vi "Periodic Tasks.vi"(8 "error in":errorcluster) -> ()   [LabVIEW 2020]
doc: "This VI runs in parallel to other tasks. It can contain as many user-defined periodic loops as you need. These can carry out PID or other sorts of timed response."
uses:
  <vilib>/Rock Robotics/WPI/ThirdParty/Phoenix-LabVIEW/Motor Controller/Controls/CTRE_Phoenix_MotorControl_TalonFXMotorControllerConfigurables.ctl
  <vilib>/Rock Robotics/WPI/ThirdParty/Phoenix-LabVIEW/Motor Controller/Controls/CTRE_Phoenix_MotorControl_BaseConfigurables.ctl
  <vilib>/Rock Robotics/WPI/ThirdParty/Phoenix-LabVIEW/Motor Controller/Controls/CTRE_Phoenix_MotorControl_VelocityMeasurementPeriod.ctl
  <vilib>/Rock Robotics/WPI/ThirdParty/Phoenix-LabVIEW/Motor Controller/Controls/CTRE_Phoenix_MotorControl_SlotStructure.ctl
  <vilib>/Rock Robotics/WPI/ThirdParty/Phoenix-LabVIEW/Motor Controller/Controls/CTRE_Phoenix_MotorControl_FilterStruct.ctl
  <vilib>/Rock Robotics/WPI/ThirdParty/Phoenix-LabVIEW/Motor Controller/Controls/CTRE_Phoenix_MotorControl_RemoteSourceType.ctl
  <vilib>/Rock Robotics/WPI/ThirdParty/Phoenix-LabVIEW/Controls/CTRE_Phoenix_CustomParamConfiguration.ctl
  <vilib>/Rock Robotics/WPI/ThirdParty/Phoenix-LabVIEW/Motor Controller/Controls/CTRE_Phoenix_MotorControl_FeedbackDevice_TalonFX.ctl
  <vilib>/Rock Robotics/WPI/ThirdParty/Phoenix-LabVIEW/Motor Controller/Controls/CTRE_Phoenix_MotorControl_LimitSwitchNormal.ctl
  <vilib>/Rock Robotics/WPI/ThirdParty/Phoenix-LabVIEW/Motor Controller/Controls/CTRE_Phoenix_MotorControl_LimitSwitchSource_Local.ctl
  <vilib>/Rock Robotics/WPI/ThirdParty/Phoenix-LabVIEW/Motor Controller/Controls/CTRE_Phoenix_MotorControl_SupplyCurrentLimitConfiguration.ctl
  <vilib>/Rock Robotics/WPI/ThirdParty/Phoenix-LabVIEW/Motor Controller/Controls/CTRE_Phoenix_MotorControl_StatorCurrentLimitConfiguration.ctl
  <vilib>/Rock Robotics/WPI/ThirdParty/Phoenix-LabVIEW/Motor Controller/Controls/CTRE_Phoenix_MotorControl_MotorCommutation_TalonFX.ctl
  <vilib>/Rock Robotics/WPI/ThirdParty/Phoenix-LabVIEW/CANCoder/Controls/CTRE_Phoenix_CANcoder_AbsoluteSensorRange.ctl
  <vilib>/Rock Robotics/WPI/ThirdParty/Phoenix-LabVIEW/CANCoder/Controls/CTRE_Phoenix_CANcoder_SensorInitializationStrategy.ctl
  <vilib>/Rock Robotics/WPI/ThirdParty/REV Robotics/REVLib/Typedef/Spark MAX Limit Direction.ctl
  <vilib>/Rock Robotics/WPI/Solenoid/WPI_SolenoidValue.ctl
  <vilib>/Rock Robotics/WPI/ThirdParty/Phoenix-LabVIEW/Motor Controller/Controls/CTRE_Phoenix_MotorControl_ControlMode.ctl
  <vilib>/Rock Robotics/WPI/DriverStation/WPI_DriverStationRobotMode2.ctl
  <vilib>/Rock Robotics/WPI/DriverStation/WPI_DriverStationAllianceInfo.ctl
  <vilib>/Rock Robotics/WPI/ThirdParty/Phoenix-LabVIEW/Motor Controller/Controls/CTRE_Phoenix_MotorControl_TalonFXInvertType.ctl
  <vilib>/Rock Robotics/WPI/ThirdParty/Phoenix-LabVIEW/Motor Controller/Controls/CTRE_Phoenix_MotorControl_NeutralMode.ctl
  <vilib>/Rock Robotics/WPI/Utilities/WPI_GetSetVariantRefNum.vi
  Robot Global Data.vi
  <vilib>/Rock Robotics/WPI/RobotDrive/WPI_RobotDriveArcadeDrive_Standard(NoSaturation).vi
  <vilib>/Rock Robotics/WPI/ThirdParty/Phoenix-LabVIEW/Motor Controller/Sensor/CTRE_Phoenix_MotorControl_SetIntegratedSensorPosition_TalonFX.vi
  <vilib>/Rock Robotics/WPI/ThirdParty/Phoenix-LabVIEW/Motor Controller/Get/CTRE_Phoenix_MotorController_GetSelectedSensorData.vi
  <vilib>/addons/control/pid/pid.llb/PID (DBL).vi
  <vilib>/Rock Robotics/WPI/Solenoid/WPI_SolenoidSetEnum.vi
  <vilib>/Rock Robotics/WPI/ThirdParty/Phoenix-LabVIEW/Motor Controller/Get/CTRE_Phoenix_MotorController_GetGeneralStatus.vi
  <vilib>/Rock Robotics/Network Tables/NT Read Number.vi
  <vilib>/Rock Robotics/Network Tables/NT Write Number.vi
  <vilib>/Rock Robotics/Network Tables/NT Write String.vi
  <vilib>/express/express arith-compare/Formula/XNode/ExpressFormulaBlockNode.xnode
  <vilib>/FRC Team #3937/Memory Library/memLib.lvlib
  <vilib>/addons/control/pid/NI_PID_pid.lvlib
panel:
  in  "DriveConfig":T1={"Base Configurables"={"openLoopRamp"=0.5, "closedLoopRamp"=0.0, "peakOutputForward"=0.7, "peakOutputReverse"=-0.7, "nominalOutputForward"=0.0, "nominalOutputReverse"=0.0, "neutralDeadband"=0.04, "voltageCompSaturation"=0.0, "voltageMeasurementFilter"=32, "velocityMeasurementPeriod"=100, "velocityMeasurementWindow"=64, "forwardSoftLimitThreshold"=0, "reverseSoftLimitThreshold"=0, "forwardSoftLimitEnable"=FALSE, "reverseSoftLimitEnable"=FALSE, "slot0"={"P"=0.0, "I"=0.0, "D"=0.0, "F"=0.0, "integralZone"=0.0, "allowableClosedLoopError"=0, "maxIntegralAccumulator"=0.0, "closedLoopPeakOutput"=1.0, "closedLoopPeriod"=1}, "slot1"={"P"=0.0, "I"=0.0, "D"=0.0, "F"=0.0, "integralZone"=0.0, "allowableClosedLoopError"=0, "maxIntegralAccumulator"=0.0, "closedLoopPeakOutput"=1.0, "closedLoopPeriod"=1}, "slot2"={"P"=0.0, "I"=0.0, "D"=0.0, "F"=0.0, "integralZone"=0.0, "allowableClosedLoopError"=0, "maxIntegralAccumulator"=0.0, "closedLoopPeakOutput"=1.0, "closedLoopPeriod"=1}, "slot3"={"P"=0.0, "I"=0.0, "D"=0.0, "F"=0.0, "integralZone"=0.0, "allowableClosedLoopError"=0, "maxIntegralAccumulator"=0.0, "closedLoopPeakOutput"=1.0, "closedLoopPeriod"=1}, "auxPIDPolarity"=FALSE, "remoteFilter0"={"remoteSensorDeviceID"=0, "remoteSensorSource"=enum."Off"}, "remoteFilter1"={"remoteSensorDeviceID"=0, "remoteSensorSource"=enum."Off"}, "motionCruiseVelocity"=0, "motionAcceleration"=0, "motionProfileTrajectoryPeriod"=0, "feedbackNotContinuous"=FALSE, "remoteSensorClosedLoopDisableNeutralOnLOS"=FALSE, "clearPositionOnLimitF"=FALSE, "clearPositionOnLimitR"=FALSE, "clearPositionOnQuadIdx"=FALSE, "limitSwitchDisableNeutralOnLOS"=FALSE, "softLimitDisableNeutralOnLOS"=FALSE, "pulseWidthPeriod_EdgesPerRot"=1, "pulseWidthPeriod_FilterWindowSz"=1, "customParam"={"customParam0"=0, "customParam1"=0}, "trajectoryInterpolationEnable"=TRUE}, "primaryPID"={"selectedFeedbackCoefficient"=1.0, "selectedFeedbackSensor"=1}, "auxiliaryPID"={"selectedFeedbackCoefficient"=1.0, "selectedFeedbackSensor"=1}, "forwardLimitSwitchNormal"=enum."Normally Open", "reverseLimitSwitchNormal"=enum."Normally Open", "forwardLimitSwitchDeviceID"=0, "reverseLimitSwitchDeviceID"=0, "forwardLimitSwitchSource"=enum."Feedback Connector", "reverseLimitSwitchSource"=enum."Feedback Connector", "sum0Term"=1, "sum1Term"=1, "diff0Term"=1, "diff1Term"=1, "Supply Current Limit Configuration"={"Enable?"=FALSE, "Current Limit"=0.0, "Threshold Current"=0.0, "Threshold Time"=0.0}, "Stator Current Limit Configuration"={"Enable?"=FALSE, "Current Limit"=0.0, "Threshold Current"=0.0, "Threshold Time"=0.0}, "Motor Commutation"=enum."Trapezoidal", "Absolute Sensor Range"=enum."Unsigned [0 to 360)", "Integrated Sensor Offset (Degrees)"=0.0, "Sensor Initialization Strategy"=enum."Boot To Zero"} {"diff1Term" items=["Integrated Sensor"=1, "Sensor Sum (S0 + S1)"=9, "Sensor Difference (D0 - D1)"=10, "Remote Source 0"=11, "Remote Source 1"=12, "None"=14, "Software Emulated"=15]; "diff0Term" items=["Integrated Sensor"=1, "Sensor Sum (S0 + S1)"=9, "Sensor Difference (D0 - D1)"=10, "Remote Source 0"=11, "Remote Source 1"=12, "None"=14, "Software Emulated"=15]; "sum1Term" items=["Integrated Sensor"=1, "Sensor Sum (S0 + S1)"=9, "Sensor Difference (D0 - D1)"=10, "Remote Source 0"=11, "Remote Source 1"=12, "None"=14, "Software Emulated"=15]; "sum0Term" items=["Integrated Sensor"=1, "Sensor Sum (S0 + S1)"=9, "Sensor Difference (D0 - D1)"=10, "Remote Source 0"=11, "Remote Source 1"=12, "None"=14, "Software Emulated"=15]; "auxiliaryPID"."selectedFeedbackSensor" items=["Integrated Sensor"=1, "Sensor Sum (S0 + S1)"=9, "Sensor Difference (D0 - D1)"=10, "Remote Source 0"=11, "Remote Source 1"=12, "None"=14, "Software Emulated"=15]; "primaryPID"."selectedFeedbackSensor" items=["Integrated Sensor"=1, "Sensor Sum (S0 + S1)"=9, "Sensor Difference (D0 - D1)"=10, "Remote Source 0"=11, "Remote Source 1"=12, "None"=14, "Software Emulated"=15]; "Base Configurables"."velocityMeasurementPeriod" items=["Period_1ms"=1, "Period_2ms"=2, "Period_5ms"=5, "Period_10ms"=10, "Period_20ms"=20, "Period_25ms"=25, "Period_50ms"=50, "Period_100ms"=100]}
  in  "ShootConfig1":T1={"Base Configurables"={"openLoopRamp"=0.0, "closedLoopRamp"=0.0, "peakOutputForward"=1.0, "peakOutputReverse"=0.0, "nominalOutputForward"=0.0, "nominalOutputReverse"=0.0, "neutralDeadband"=0.04, "voltageCompSaturation"=0.0, "voltageMeasurementFilter"=32, "velocityMeasurementPeriod"=100, "velocityMeasurementWindow"=64, "forwardSoftLimitThreshold"=0, "reverseSoftLimitThreshold"=0, "forwardSoftLimitEnable"=FALSE, "reverseSoftLimitEnable"=FALSE, "slot0"={"P"=0.32, "I"=0.0, "D"=45.0, "F"=0.047, "integralZone"=0.0, "allowableClosedLoopError"=0, "maxIntegralAccumulator"=0.0, "closedLoopPeakOutput"=1.0, "closedLoopPeriod"=1}, "slot1"={"P"=0.0, "I"=0.0, "D"=0.0, "F"=0.0, "integralZone"=0.0, "allowableClosedLoopError"=0, "maxIntegralAccumulator"=0.0, "closedLoopPeakOutput"=1.0, "closedLoopPeriod"=1}, "slot2"={"P"=0.0, "I"=0.0, "D"=0.0, "F"=0.0, "integralZone"=0.0, "allowableClosedLoopError"=0, "maxIntegralAccumulator"=0.0, "closedLoopPeakOutput"=1.0, "closedLoopPeriod"=1}, "slot3"={"P"=0.0, "I"=0.0, "D"=0.0, "F"=0.0, "integralZone"=0.0, "allowableClosedLoopError"=0, "maxIntegralAccumulator"=0.0, "closedLoopPeakOutput"=1.0, "closedLoopPeriod"=1}, "auxPIDPolarity"=FALSE, "remoteFilter0"={"remoteSensorDeviceID"=0, "remoteSensorSource"=enum."Off"}, "remoteFilter1"={"remoteSensorDeviceID"=0, "remoteSensorSource"=enum."Off"}, "motionCruiseVelocity"=0, "motionAcceleration"=0, "motionProfileTrajectoryPeriod"=0, "feedbackNotContinuous"=FALSE, "remoteSensorClosedLoopDisableNeutralOnLOS"=FALSE, "clearPositionOnLimitF"=FALSE, "clearPositionOnLimitR"=FALSE, "clearPositionOnQuadIdx"=FALSE, "limitSwitchDisableNeutralOnLOS"=FALSE, "softLimitDisableNeutralOnLOS"=FALSE, "pulseWidthPeriod_EdgesPerRot"=1, "pulseWidthPeriod_FilterWindowSz"=1, "customParam"={"customParam0"=0, "customParam1"=0}, "trajectoryInterpolationEnable"=TRUE}, "primaryPID"={"selectedFeedbackCoefficient"=1.0, "selectedFeedbackSensor"=1}, "auxiliaryPID"={"selectedFeedbackCoefficient"=1.0, "selectedFeedbackSensor"=1}, "forwardLimitSwitchNormal"=enum."Normally Open", "reverseLimitSwitchNormal"=enum."Normally Open", "forwardLimitSwitchDeviceID"=0, "reverseLimitSwitchDeviceID"=0, "forwardLimitSwitchSource"=enum."Feedback Connector", "reverseLimitSwitchSource"=enum."Feedback Connector", "sum0Term"=1, "sum1Term"=1, "diff0Term"=1, "diff1Term"=1, "Supply Current Limit Configuration"={"Enable?"=FALSE, "Current Limit"=0.0, "Threshold Current"=0.0, "Threshold Time"=0.0}, "Stator Current Limit Configuration"={"Enable?"=FALSE, "Current Limit"=0.0, "Threshold Current"=0.0, "Threshold Time"=0.0}, "Motor Commutation"=enum."Trapezoidal", "Absolute Sensor Range"=enum."Unsigned [0 to 360)", "Integrated Sensor Offset (Degrees)"=0.0, "Sensor Initialization Strategy"=enum."Boot To Zero"} {"diff1Term" items=["Integrated Sensor"=1, "Sensor Sum (S0 + S1)"=9, "Sensor Difference (D0 - D1)"=10, "Remote Source 0"=11, "Remote Source 1"=12, "None"=14, "Software Emulated"=15]; "diff0Term" items=["Integrated Sensor"=1, "Sensor Sum (S0 + S1)"=9, "Sensor Difference (D0 - D1)"=10, "Remote Source 0"=11, "Remote Source 1"=12, "None"=14, "Software Emulated"=15]; "sum1Term" items=["Integrated Sensor"=1, "Sensor Sum (S0 + S1)"=9, "Sensor Difference (D0 - D1)"=10, "Remote Source 0"=11, "Remote Source 1"=12, "None"=14, "Software Emulated"=15]; "sum0Term" items=["Integrated Sensor"=1, "Sensor Sum (S0 + S1)"=9, "Sensor Difference (D0 - D1)"=10, "Remote Source 0"=11, "Remote Source 1"=12, "None"=14, "Software Emulated"=15]; "auxiliaryPID"."selectedFeedbackSensor" items=["Integrated Sensor"=1, "Sensor Sum (S0 + S1)"=9, "Sensor Difference (D0 - D1)"=10, "Remote Source 0"=11, "Remote Source 1"=12, "None"=14, "Software Emulated"=15]; "primaryPID"."selectedFeedbackSensor" items=["Integrated Sensor"=1, "Sensor Sum (S0 + S1)"=9, "Sensor Difference (D0 - D1)"=10, "Remote Source 0"=11, "Remote Source 1"=12, "None"=14, "Software Emulated"=15]; "Base Configurables"."velocityMeasurementPeriod" items=["Period_1ms"=1, "Period_2ms"=2, "Period_5ms"=5, "Period_10ms"=10, "Period_20ms"=20, "Period_25ms"=25, "Period_50ms"=50, "Period_100ms"=100]}
  in  "ShootConfig2":T1={"Base Configurables"={"openLoopRamp"=0.0, "closedLoopRamp"=0.0, "peakOutputForward"=1.0, "peakOutputReverse"=0.0, "nominalOutputForward"=0.0, "nominalOutputReverse"=0.0, "neutralDeadband"=0.04, "voltageCompSaturation"=0.0, "voltageMeasurementFilter"=32, "velocityMeasurementPeriod"=100, "velocityMeasurementWindow"=64, "forwardSoftLimitThreshold"=0, "reverseSoftLimitThreshold"=0, "forwardSoftLimitEnable"=FALSE, "reverseSoftLimitEnable"=FALSE, "slot0"={"P"=0.32, "I"=0.0, "D"=45.0, "F"=0.0475, "integralZone"=0.0, "allowableClosedLoopError"=0, "maxIntegralAccumulator"=0.0, "closedLoopPeakOutput"=1.0, "closedLoopPeriod"=1}, "slot1"={"P"=0.0, "I"=0.0, "D"=0.0, "F"=0.0, "integralZone"=0.0, "allowableClosedLoopError"=0, "maxIntegralAccumulator"=0.0, "closedLoopPeakOutput"=1.0, "closedLoopPeriod"=1}, "slot2"={"P"=0.0, "I"=0.0, "D"=0.0, "F"=0.0, "integralZone"=0.0, "allowableClosedLoopError"=0, "maxIntegralAccumulator"=0.0, "closedLoopPeakOutput"=1.0, "closedLoopPeriod"=1}, "slot3"={"P"=0.0, "I"=0.0, "D"=0.0, "F"=0.0, "integralZone"=0.0, "allowableClosedLoopError"=0, "maxIntegralAccumulator"=0.0, "closedLoopPeakOutput"=1.0, "closedLoopPeriod"=1}, "auxPIDPolarity"=FALSE, "remoteFilter0"={"remoteSensorDeviceID"=0, "remoteSensorSource"=enum."Off"}, "remoteFilter1"={"remoteSensorDeviceID"=0, "remoteSensorSource"=enum."Off"}, "motionCruiseVelocity"=0, "motionAcceleration"=0, "motionProfileTrajectoryPeriod"=0, "feedbackNotContinuous"=FALSE, "remoteSensorClosedLoopDisableNeutralOnLOS"=FALSE, "clearPositionOnLimitF"=FALSE, "clearPositionOnLimitR"=FALSE, "clearPositionOnQuadIdx"=FALSE, "limitSwitchDisableNeutralOnLOS"=FALSE, "softLimitDisableNeutralOnLOS"=FALSE, "pulseWidthPeriod_EdgesPerRot"=1, "pulseWidthPeriod_FilterWindowSz"=1, "customParam"={"customParam0"=0, "customParam1"=0}, "trajectoryInterpolationEnable"=TRUE}, "primaryPID"={"selectedFeedbackCoefficient"=1.0, "selectedFeedbackSensor"=1}, "auxiliaryPID"={"selectedFeedbackCoefficient"=1.0, "selectedFeedbackSensor"=1}, "forwardLimitSwitchNormal"=enum."Normally Open", "reverseLimitSwitchNormal"=enum."Normally Open", "forwardLimitSwitchDeviceID"=0, "reverseLimitSwitchDeviceID"=0, "forwardLimitSwitchSource"=enum."Feedback Connector", "reverseLimitSwitchSource"=enum."Feedback Connector", "sum0Term"=1, "sum1Term"=1, "diff0Term"=1, "diff1Term"=1, "Supply Current Limit Configuration"={"Enable?"=FALSE, "Current Limit"=0.0, "Threshold Current"=0.0, "Threshold Time"=0.0}, "Stator Current Limit Configuration"={"Enable?"=FALSE, "Current Limit"=0.0, "Threshold Current"=0.0, "Threshold Time"=0.0}, "Motor Commutation"=enum."Trapezoidal", "Absolute Sensor Range"=enum."Unsigned [0 to 360)", "Integrated Sensor Offset (Degrees)"=0.0, "Sensor Initialization Strategy"=enum."Boot To Zero"} {"diff1Term" items=["Integrated Sensor"=1, "Sensor Sum (S0 + S1)"=9, "Sensor Difference (D0 - D1)"=10, "Remote Source 0"=11, "Remote Source 1"=12, "None"=14, "Software Emulated"=15]; "diff0Term" items=["Integrated Sensor"=1, "Sensor Sum (S0 + S1)"=9, "Sensor Difference (D0 - D1)"=10, "Remote Source 0"=11, "Remote Source 1"=12, "None"=14, "Software Emulated"=15]; "sum1Term" items=["Integrated Sensor"=1, "Sensor Sum (S0 + S1)"=9, "Sensor Difference (D0 - D1)"=10, "Remote Source 0"=11, "Remote Source 1"=12, "None"=14, "Software Emulated"=15]; "sum0Term" items=["Integrated Sensor"=1, "Sensor Sum (S0 + S1)"=9, "Sensor Difference (D0 - D1)"=10, "Remote Source 0"=11, "Remote Source 1"=12, "None"=14, "Software Emulated"=15]; "auxiliaryPID"."selectedFeedbackSensor" items=["Integrated Sensor"=1, "Sensor Sum (S0 + S1)"=9, "Sensor Difference (D0 - D1)"=10, "Remote Source 0"=11, "Remote Source 1"=12, "None"=14, "Software Emulated"=15]; "primaryPID"."selectedFeedbackSensor" items=["Integrated Sensor"=1, "Sensor Sum (S0 + S1)"=9, "Sensor Difference (D0 - D1)"=10, "Remote Source 0"=11, "Remote Source 1"=12, "None"=14, "Software Emulated"=15]; "Base Configurables"."velocityMeasurementPeriod" items=["Period_1ms"=1, "Period_2ms"=2, "Period_5ms"=5, "Period_10ms"=10, "Period_20ms"=20, "Period_25ms"=25, "Period_50ms"=50, "Period_100ms"=100]}
  # "Sum and Diff terms are ways to select more than one sensor as a feedback device. \n Sum 0 is the first feedback device to be used for the Sum term.\n Sum 1 is the feedback device to be added to Sum 0 for the Sum term.\n Diff 0 and Diff 1 work in a similar manner."
  # "These are only applicable\nif using a remote limit switch.\n\nLocal limit switches/no limit\nswitches do not use this."
  # "Current is below Current Limit AND\n\n(Requested output is weaker** than applied motor\noutput OR is in the opposite direction).\n/\nMotor output is set to requested output."
  # "Current is above Threshold Current for Threshold Time\n/\nReduce motor output (towards neutral)."
  # "Current is below Current Limit.\n/\nRamp motor output towards requested output."
  # "Current is above Current Limit.\n/\nReduce motor output (towards neutral)."
  # "*If the configured Peak Threshold is less than the Continuous Threshold, the applied Peak Threshold is set equal to the Configured Continuous Threshold in firmware.\n** Both requested output and applied motor output are in the same direction, and requested output is closer to neutral."
  # "False: Primary Output = PID[0] + PID[1]  ---  Auxiliary Output = PID[0] - PID[1]\nTrue:  Primary Output = PID[0] - PID[1] --- Auxiliary Output = PID[0] + PID[1]"
  # "Enable the motion profile executor to perform linear interpolation between profile points.  Defaults to True."
  # "Sum and Diff terms are ways to select more than one sensor as a feedback device. \n Sum 0 is the first feedback device to be used for the Sum term.\n Sum 1 is the feedback device to be added to Sum 0 for the Sum term.\n Diff 0 and Diff 1 work in a similar manner."
  # "These are only applicable\nif using a remote limit switch.\n\nLocal limit switches/no limit\nswitches do not use this."
  # "Current is below Current Limit AND\n\n(Requested output is weaker** than applied motor\noutput OR is in the opposite direction).\n/\nMotor output is set to requested output."
  # "Current is above Threshold Current for Threshold Time\n/\nReduce motor output (towards neutral)."
  # "Current is below Current Limit.\n/\nRamp motor output towards requested output."
  # "Current is above Current Limit.\n/\nReduce motor output (towards neutral)."
  # "*If the configured Peak Threshold is less than the Continuous Threshold, the applied Peak Threshold is set equal to the Configured Continuous Threshold in firmware.\n** Both requested output and applied motor output are in the same direction, and requested output is closer to neutral."
  # "False: Primary Output = PID[0] + PID[1]  ---  Auxiliary Output = PID[0] - PID[1]\nTrue:  Primary Output = PID[0] - PID[1] --- Auxiliary Output = PID[0] + PID[1]"
  # "Enable the motion profile executor to perform linear interpolation between profile points.  Defaults to True."
  # "Sum and Diff terms are ways to select more than one sensor as a feedback device. \n Sum 0 is the first feedback device to be used for the Sum term.\n Sum 1 is the feedback device to be added to Sum 0 for the Sum term.\n Diff 0 and Diff 1 work in a similar manner."
  # "These are only applicable\nif using a remote limit switch.\n\nLocal limit switches/no limit\nswitches do not use this."
  # "Current is below Current Limit AND\n\n(Requested output is weaker** than applied motor\noutput OR is in the opposite direction).\n/\nMotor output is set to requested output."
  # "Current is above Threshold Current for Threshold Time\n/\nReduce motor output (towards neutral)."
  # "Current is below Current Limit.\n/\nRamp motor output towards requested output."
  # "Current is above Current Limit.\n/\nReduce motor output (towards neutral)."
  # "*If the configured Peak Threshold is less than the Continuous Threshold, the applied Peak Threshold is set equal to the Configured Continuous Threshold in firmware.\n** Both requested output and applied motor output are in the same direction, and requested output is closer to neutral."
  # "False: Primary Output = PID[0] + PID[1]  ---  Auxiliary Output = PID[0] - PID[1]\nTrue:  Primary Output = PID[0] - PID[1] --- Auxiliary Output = PID[0] + PID[1]"
  # "Enable the motion profile executor to perform linear interpolation between profile points.  Defaults to True."
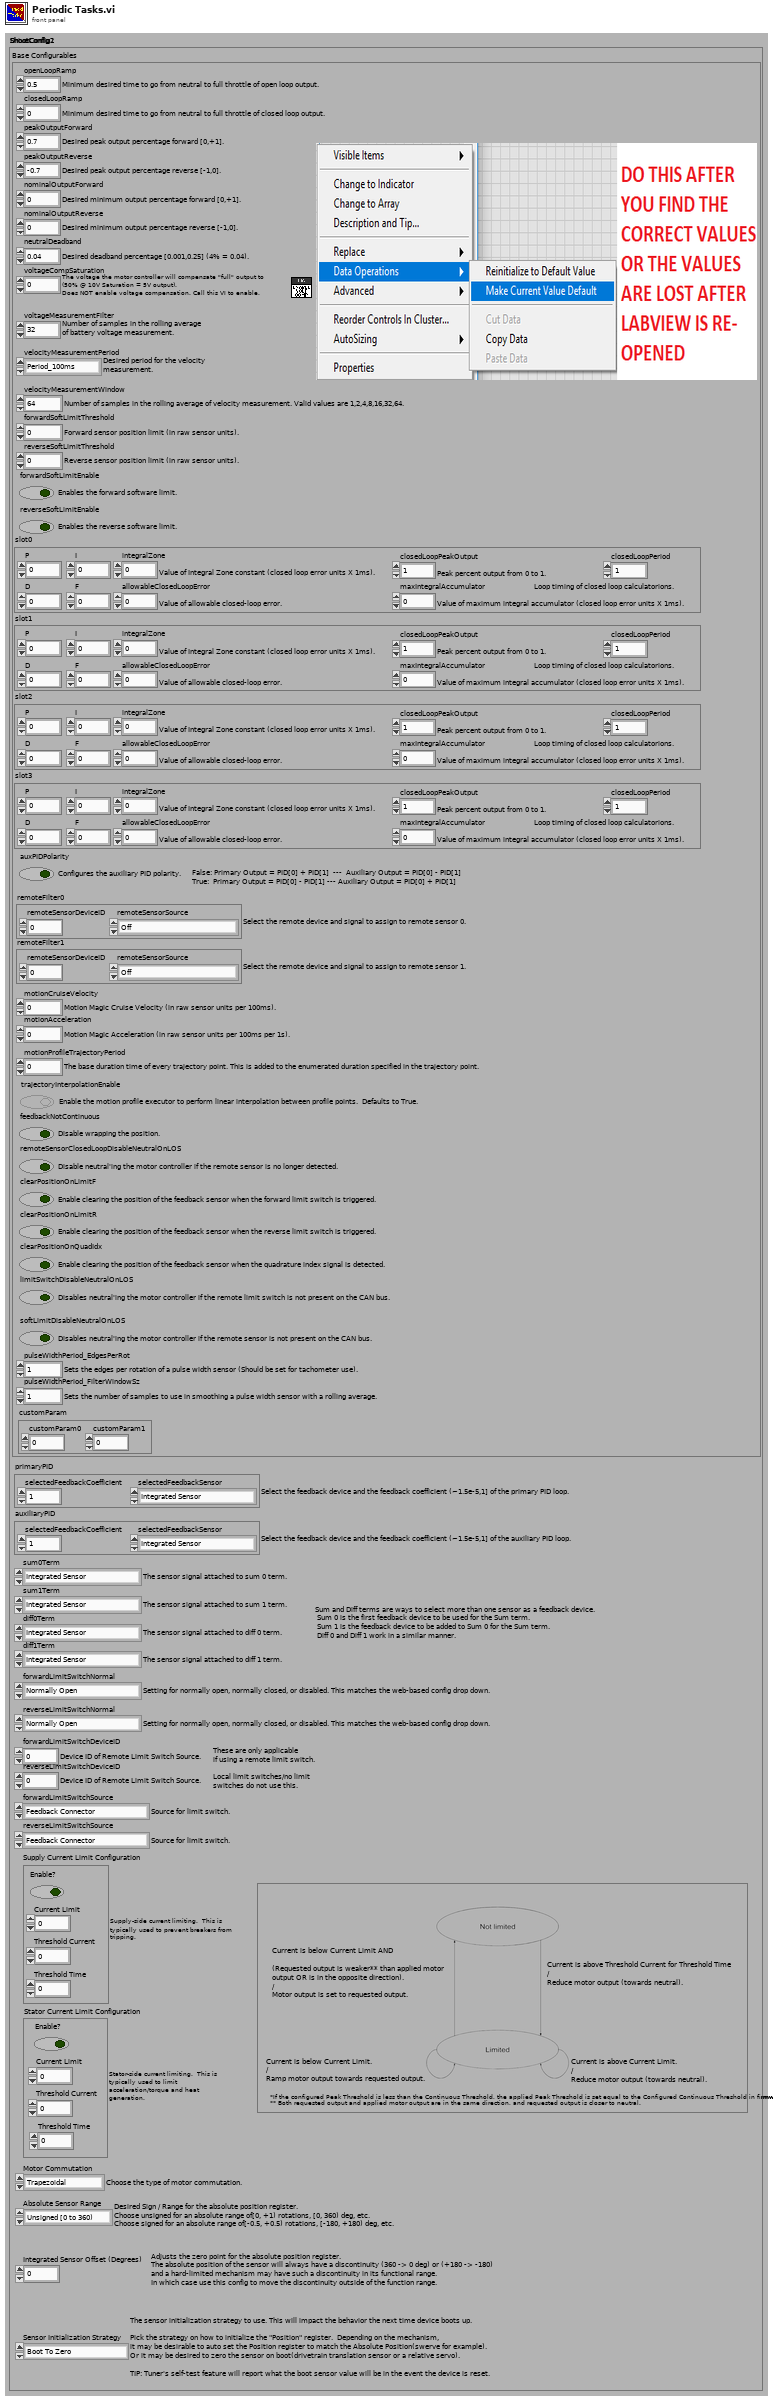
[diagram p1: front panel]
types:
  T1 = typedef "CTRE_Phoenix_MotorControl_TalonFXMotorControllerConfigurables.ctl" = cluster{"Base Configurables":T2, "primaryPID":cluster{"selectedFeedbackCoefficient":dbl, "selectedFeedbackSensor":T8}, "auxiliaryPID":cluster{"selectedFeedbackCoefficient":dbl, "selectedFeedbackSensor":T8}, "forwardLimitSwitchNormal":T9, "reverseLimitSwitchNormal":T9, "forwardLimitSwitchDeviceID":i32, "reverseLimitSwitchDeviceID":i32, "forwardLimitSwitchSource":T10, "reverseLimitSwitchSource":T10, "sum0Term":T8, "sum1Term":T8, "diff0Term":T8, "diff1Term":T8, "Supply Current Limit Configuration":T11, "Stator Current Limit Configuration":T12, "Motor Commutation":T13, "Absolute Sensor Range":T14, "Integrated Sensor Offset (Degrees)":dbl, "Sensor Initialization Strategy":T15}
  T2 = typedef "CTRE_Phoenix_MotorControl_BaseConfigurables.ctl" = cluster{"openLoopRamp":dbl, "closedLoopRamp":dbl, "peakOutputForward":dbl, "peakOutputReverse":dbl, "nominalOutputForward":dbl, "nominalOutputReverse":dbl, "neutralDeadband":dbl, "voltageCompSaturation":dbl, "voltageMeasurementFilter":i32, "velocityMeasurementPeriod":T3, "velocityMeasurementWindow":i32, "forwardSoftLimitThreshold":i32, "reverseSoftLimitThreshold":i32, "forwardSoftLimitEnable":bool, "reverseSoftLimitEnable":bool, "slot0":T4, "slot1":T4, "slot2":T4, "slot3":T4, "auxPIDPolarity":bool, "remoteFilter0":T5, "remoteFilter1":T5, "motionCruiseVelocity":i32, "motionAcceleration":i32, "motionProfileTrajectoryPeriod":i32, "feedbackNotContinuous":bool, "remoteSensorClosedLoopDisableNeutralOnLOS":bool, "clearPositionOnLimitF":bool, "clearPositionOnLimitR":bool, "clearPositionOnQuadIdx":bool, "limitSwitchDisableNeutralOnLOS":bool, "softLimitDisableNeutralOnLOS":bool, "pulseWidthPeriod_EdgesPerRot":i32, "pulseWidthPeriod_FilterWindowSz":i32, "customParam":T7, "trajectoryInterpolationEnable":bool}
  T3 = typedef "CTRE_Phoenix_MotorControl_VelocityMeasurementPeriod.ctl" = u16
  T4 = typedef "CTRE_Phoenix_MotorControl_SlotStructure.ctl" = cluster{"P":dbl, "I":dbl, "D":dbl, "F":dbl, "integralZone":dbl, "allowableClosedLoopError":i32, "maxIntegralAccumulator":dbl, "closedLoopPeakOutput":dbl, "closedLoopPeriod":i32}
  T5 = typedef "CTRE_Phoenix_MotorControl_FilterStruct.ctl" = cluster{"remoteSensorDeviceID":u8, "remoteSensorSource":T6}
  T6 = typedef "CTRE_Phoenix_MotorControl_RemoteSourceType.ctl" = enum16{"Off", "Talon SRX Selected Sensor", "Pigeon IMU Yaw", "Pigeon IMU Pitch", "Pigeon IMU Roll", "CANifier Quadrature", "CANifier PWM Input 0", "CANifier PWM Input 1", "CANifier PWM Input 2", "CANifier PWM Input 3", "Gadgeteer Pigeon Yaw", "Gadgeteer Pigeon Pitch", "Gadgeteer Pigeon Roll", "CANCoder"}
  T7 = typedef "CTRE_Phoenix_CustomParamConfiguration.ctl" = cluster{"customParam0":i32, "customParam1":i32}
  T8 = typedef "CTRE_Phoenix_MotorControl_FeedbackDevice_TalonFX.ctl" = i8
  T9 = typedef "CTRE_Phoenix_MotorControl_LimitSwitchNormal.ctl" = enum16{"Normally Open", "Normally Closed", "Disabled"}
  T10 = typedef "CTRE_Phoenix_MotorControl_LimitSwitchSource_Local.ctl" = enum16{"Feedback Connector", "Remote Talon SRX", "Remote CANifier", "Deactivated"}
  T11 = typedef "CTRE_Phoenix_MotorControl_SupplyCurrentLimitConfiguration.ctl" = cluster{"Enable?":bool, "Current Limit":dbl, "Threshold Current":dbl, "Threshold Time":dbl}
  T12 = typedef "CTRE_Phoenix_MotorControl_StatorCurrentLimitConfiguration.ctl" = cluster{"Enable?":bool, "Current Limit":dbl, "Threshold Current":dbl, "Threshold Time":dbl}
  T13 = typedef "CTRE_Phoenix_MotorControl_MotorCommutation_TalonFX.ctl" = enum16{"Trapezoidal"}
  T14 = typedef "CTRE_Phoenix_CANcoder_AbsoluteSensorRange.ctl" = enum16{"Unsigned [0 to 360)", "Signed [-180 to +180)"}
  T15 = typedef "CTRE_Phoenix_CANcoder_SensorInitializationStrategy.ctl" = enum16{"Boot To Zero", "Boot To Absolute Position"}
  T16 = enum16{"Initialize", "Wait", "Extend", "Midbar", "FlipOn", "UnClimb"}
  T17 = enum16{"Initialize", "Wait", "LowShot", "HighShot", "AutoShot"}
  T18 = typedef "Spark MAX Limit Direction.ctl" = enum16{"Forward Limit", "Reverse Limit"}
  T19 = enum16{"Initialize", "Manual", "PID", "AutoCenter"}
  T20 = typedef "WPI_MotorControlDeviceRef.ctl" = cluster{"DeviceStatus":errorcluster, "Type":T21, "PWM":cluster{"PWM Channel":T22, "DeadBand":T23}, "CAN":cluster{"Device Number":u8, "SetOutput VI Ref":variant, "GetOutput VI Ref":variant, "Enable VI Ref":variant, "Disable VI Ref":variant, "Data":variant}, "Invert":bool, "DIO PWM":cluster{"PWM \"Enable\" Channel":T22, "DIOChannel":T24, "PWM Rate":dbl}}
  T21 = typedef "WPI_MotorControlType.ctl" = enum16{"PWM", "CAN", "DIO PWM"}
  T22 = typedef "FPGA_DIOPWMChannel.ctl" = enum8{"PWM 0", "PWM 1", "PWM 2", "PWM 3", "PWM 4", "PWM 5", "PWM 6", "PWM 7", "PWM 8", "PWM 9", "PWM MXP 0", "PWM MXP 1", "PWM MXP 2", "PWM MXP 3", "PWM MXP 4", "PWM MXP 5", "PWM MXP 6", "PWM MXP 7", "PWM MXP 8", "PWM MXP 9", "Invalid"}
  T23 = typedef "WPI_PWMDeadband.ctl" = cluster{"Name":string, "maxPositivePwm":i32, "minPositivePwm":i32, "centerPwm":i32, "maxNegativePwm":i32, "minNegativePwm":i32, "angularRange":u16}
  T24 = typedef "FPGA_DIOChannel.ctl" = enum8{"DIO 0", "DIO 1", "DIO 2", "DIO 3", "DIO 4", "DIO 5", "DIO 6", "DIO 7", "DIO 8", "DIO 9", "DIO MXP 0", "DIO MXP 1", "DIO MXP 2", "DIO MXP 3", "DIO MXP 4", "DIO MXP 5", "DIO MXP 6", "DIO MXP 7", "DIO MXP 8", "DIO MXP 9", "DIO MXP 10", "DIO MXP 11", "DIO MXP 12", "DIO MXP 13", "DIO MXP 14", "DIO MXP 15", "SPI Port CS1", "SPI Port CS2", "SPI Port CS3", "SPI Port MISO", "SPI Port MOSI", "Invalid"}
  T25 = typedef "CTRE_Phoenix_MotorControl_NeutralMode.ctl" = enum8{"EEPROMSetting", "Override to Coast", "Override to Brake"}
  T26 = typedef "CTRE_Phoenix_MotorControl_TalonFXInvertType.ctl" = enum16{"Counter-Clockwise", "Clockwise"}
  T27 = typedef "CTRE_Phoenix_MotorControl_ControlMode.ctl" = u16
  T28 = typedef "WPI_SolenoidDevRef.ctl" = cluster{"DevStatus":errorcluster, "Pneumatics Control Module":u8, "Forward Solenoid Channel":T29, "Reverse Solenoid Channel":T29}
  T29 = typedef "WPI_SolenoidChannel.ctl" = enum8{"Solenoid 0", "Solenoid 1", "Solenoid 2", "Solenoid 3", "Solenoid 4", "Solenoid 5", "Solenoid 6", "Solenoid 7", "Solenoid 8", "Solenoid 9", "Solenoid 10", "Solenoid 11", "Solenoid 12", "Solenoid 13", "Solenoid 14", "Solenoid 15", "Invalid"}
  T30 = typedef "WPI_RobotDriveDevRef.ctl" = cluster{"DevStatus":errorcluster, "Motors[]":T20[], "Square Inputs":bool, "Max Output":dbl}
  T31 = typedef "WPI_SolenoidValue.ctl" = enum16{"Off", "On", "Forward", "Reverse"}
  T32 = cluster{"proportional gain (Kp)":dbl, "integral time (Ki)":dbl, "derivative time (Kd)":dbl}
  T33 = typedef "ADIS16470 Device Reference.ctl" = cluster{"DevStatus":errorcluster, "Hardware Config":T34, "Calibration Complete":refnum<notifier>, "Status FIFO":refnum<k33>, "Last Value Reference":refnum<data-value>, "Sychronous Process VI":T37, "Cmd FIFO":refnum<k33>, "Source":T38, "Data FIFO":refnum<k33>, "Calibration Time":T42}
  T34 = typedef "ADIS16470 Hardware Configuration.ctl" = cluster{"SPI Clock Rate (Hz)":dbl, "IMU SPI Mode (3)":T35, "IMU Reset Pin":T24, "IMU SPI Bus":T36, "IMU Data Ready Pin":T24, "Stall Config":cluster{"Pow2BytesPerRead":u8, "StallTicks":u16, "CsToSclkTicks":u8}}
  T35 = typedef "WPI_SPIMode.ctl" = enum16{"Mode 0 (Clk Idle Low,Sample on Leading)", "Mode 1 (Clk Idle Low,Sample on Trailing)", "Mode 2 (Clk Idle High,Sample on Leading)", "Mode 3 (Clk Idle High,Sample on Trailing)"}
  T36 = typedef "spi_bus.ctl" = enum16{"SPI On-Board, CS0", "SPI On-Board, CS1", "SPI On-Board, CS2", "SPI On-Board, CS3", "SPI MXP", "Invalid"}
  T37 = typedef "ADIS16470 Process.ctl" = refnum<vi>
  T38 = typedef "FPGA_CounterEncoderSourceConvertionLVSourceType.ctl" = cluster{"DevStatus":errorcluster, "AnalogTriggerMode?":bool, "DigitalMode":cluster{"DIO Channel":T39}, "AnalogTriggerMode":cluster{"AnalogTriggerIndex":T40, "OutputType":T41}}
  T39 = typedef "FPGA_DIODigitalSourceChannel.ctl" = enum8{"DIO 0", "DIO 1", "DIO 2", "DIO 3", "DIO 4", "DIO 5", "DIO 6", "DIO 7", "DIO 8", "DIO 9", "DIO MXP 0", "DIO MXP 1", "DIO MXP 2", "DIO MXP 3", "DIO MXP 4", "DIO MXP 5", "DIO MXP 6", "DIO MXP 7", "DIO MXP 8", "DIO MXP 9", "DIO MXP 10", "DIO MXP 11", "DIO MXP 12", "DIO MXP 13", "DIO MXP 14", "DIO MXP 15", "SPI Port CS1", "SPI Port CS2", "SPI Port CS3", "SPI Port MISO", "SPI Port MOSI", "Disabled"}
  T40 = typedef "FPGA_AnalogTriggerIndex.ctl" = enum8{"Trig 0", "Trig 1", "Trig 2", "Trig 3", "Trig 4", "Trig 5", "Trig 6", "Trig 7", "Invalid"}
  T41 = typedef "FPGA_AnalogTriggerOutType.ctl" = enum16{"InWindow", "TriggerState", "Rising", "Falling"}
  T42 = typedef "ADIS16470 Calibration Time.ctl" = enum16{"32ms", "64ms", "128ms", "256ms", "512ms", "1s", "2s", "4s", "8s", "16s", "32s", "64s"}
  T43 = typedef "WPI_DriverStationAllianceInfo.ctl" = enum16{"Red", "Blue", "Invalid"}
  T44 = typedef "ADIS16470 Data.ctl" = cluster{"XAngle":dbl, "YAngle":dbl, "ZAngle":dbl}
  T45 = typedef "WPI_DriverStationRobotMode2.ctl" = enum16{"Autonomous Disabled", "Autonomous Enabled", "Teleop Disabled", "Teleop Enabled", "Disconnected", "Finish", "Test Disabled", "Test Enabled", "Emergency Stopped"}
  T46 = typedef "WPI_CompressorDevRef.ctl" = cluster{"DevStatus":errorcluster, "Pneumatics Control Module":u8}
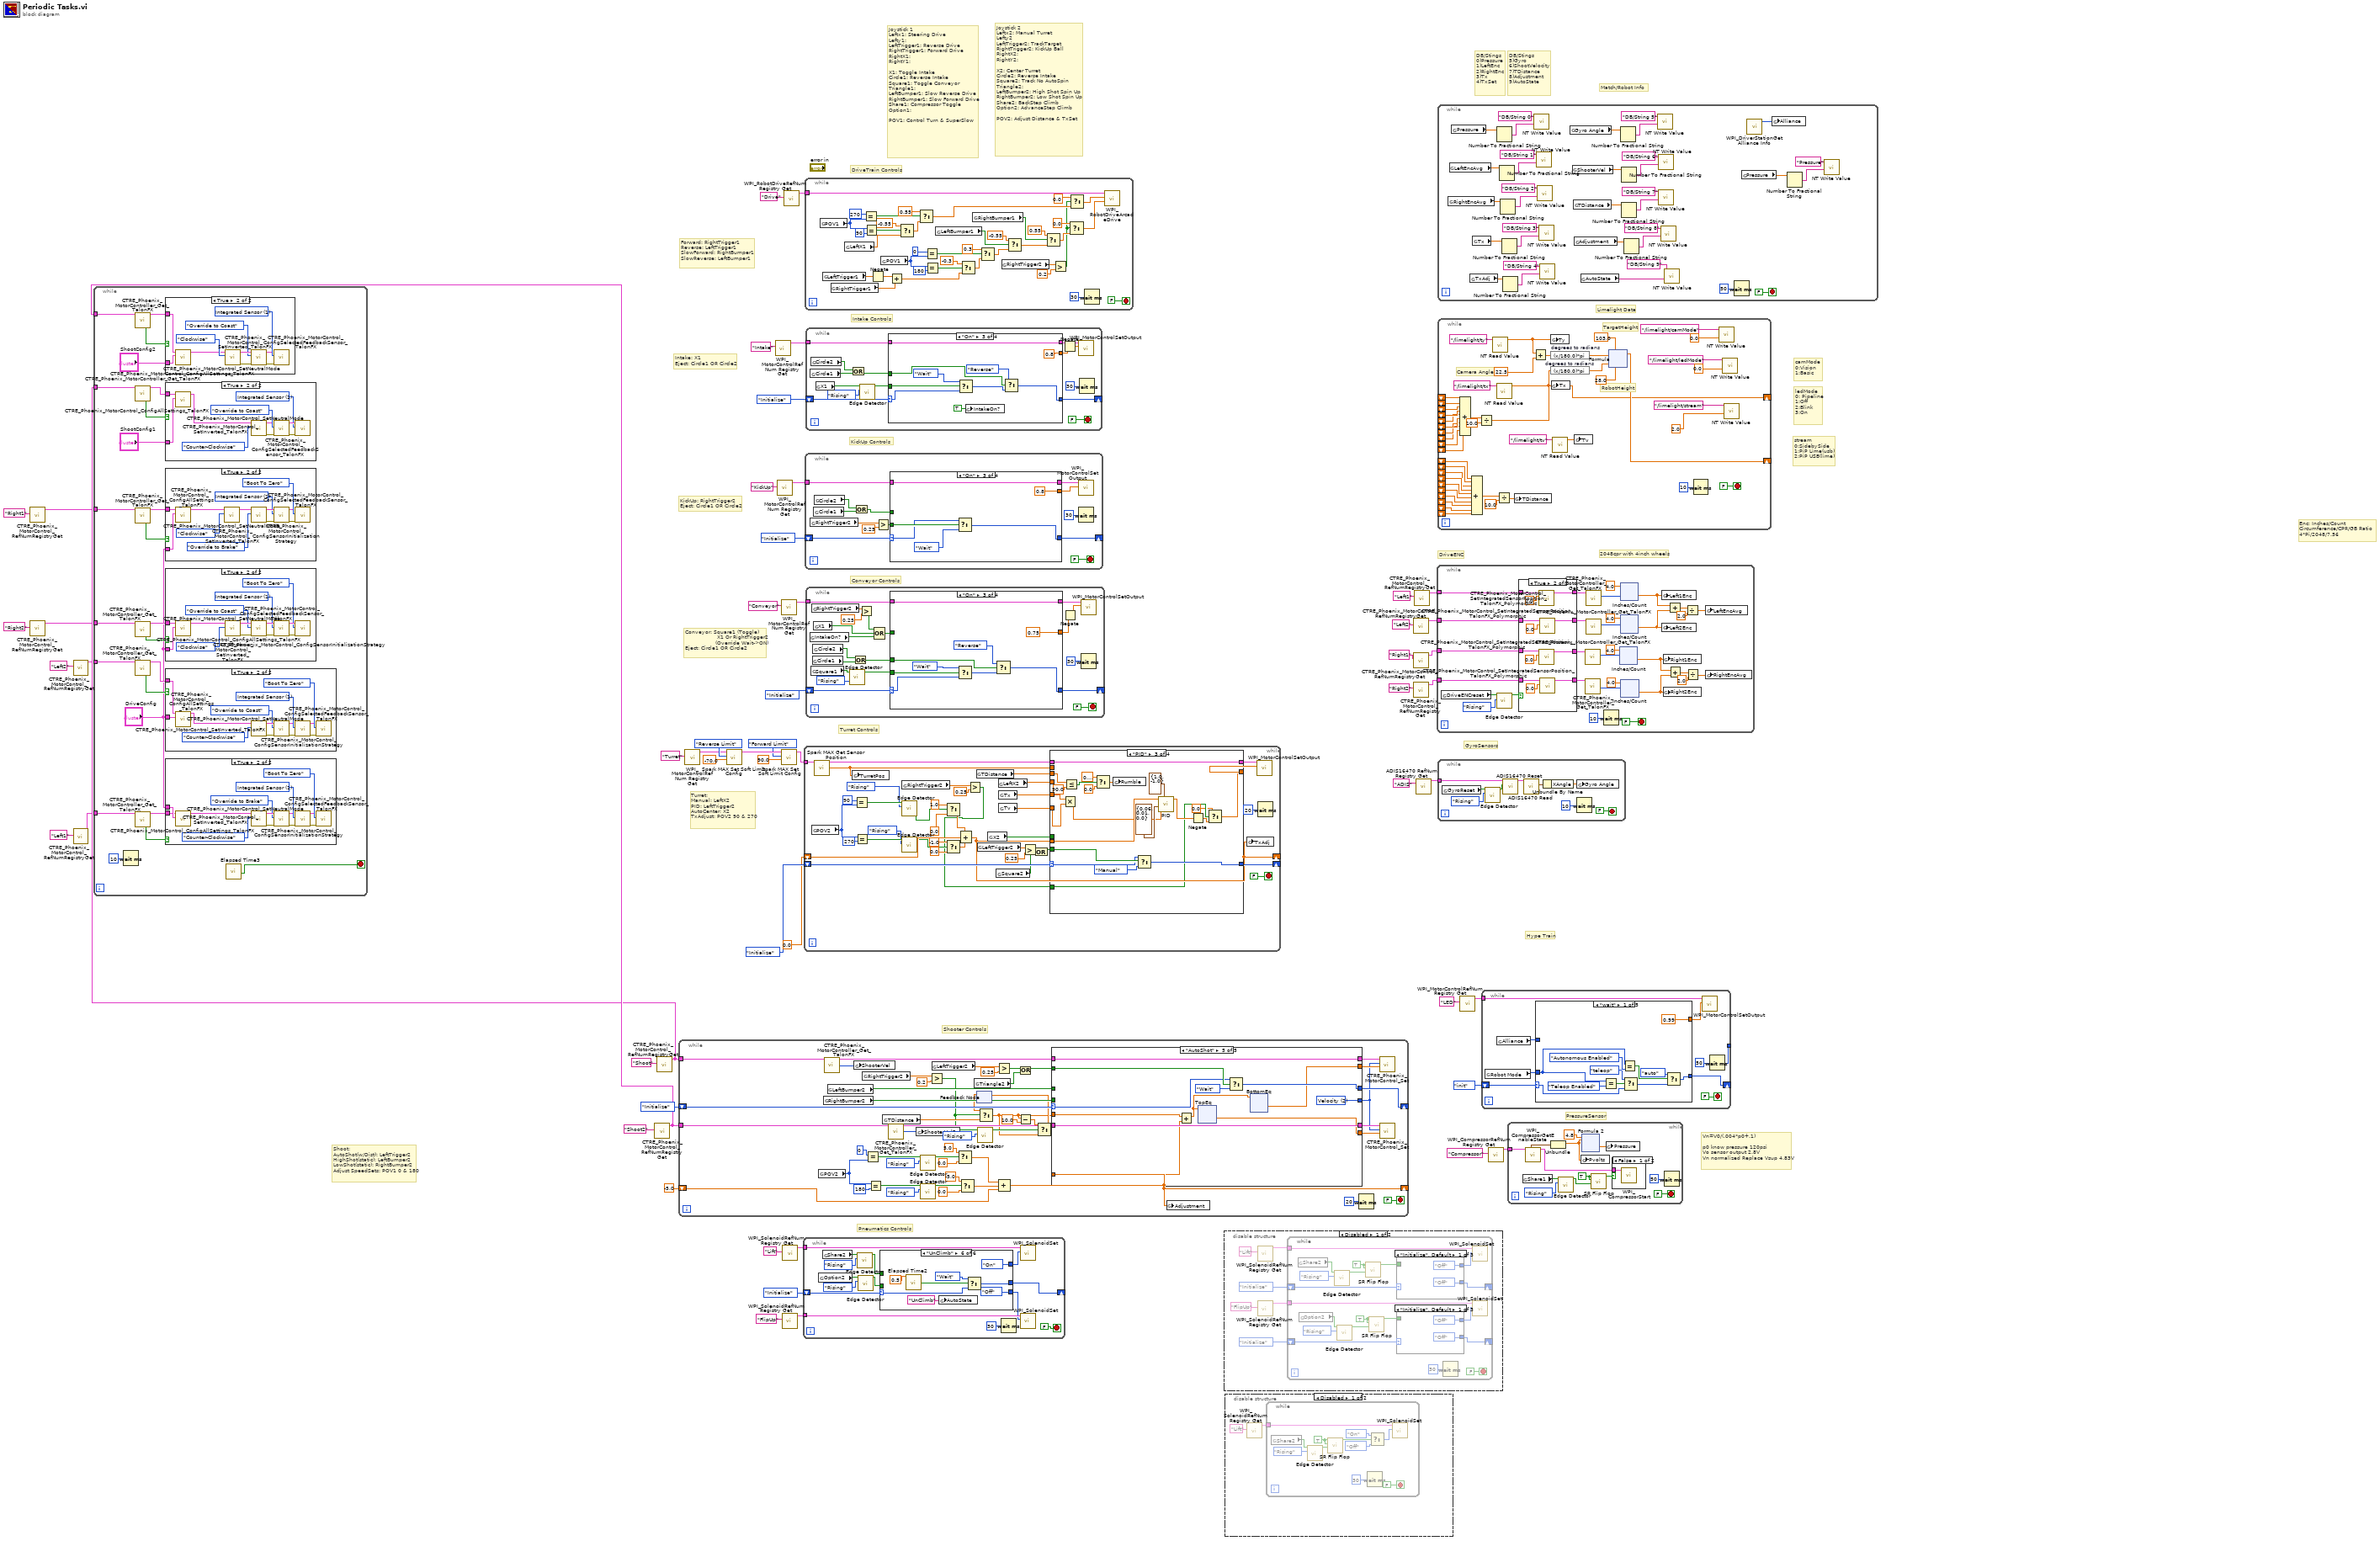
[diagram p0: block diagram]
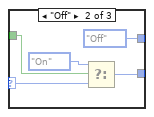
[diagram p8: hidden frame]
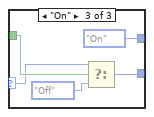
[diagram p9: hidden frame]
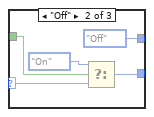
[diagram p10: hidden frame]
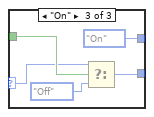
[diagram p11: hidden frame]
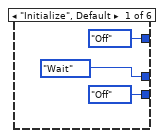
[diagram p13: hidden frame]
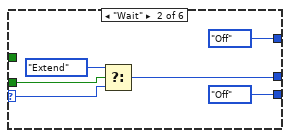
[diagram p14: hidden frame]
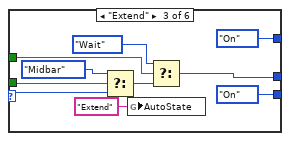
[diagram p15: hidden frame]
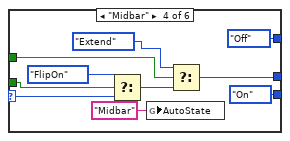
[diagram p16: hidden frame]
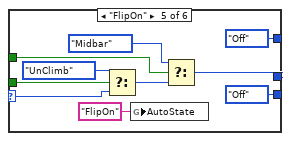
[diagram p17: hidden frame]
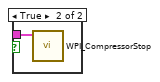
[diagram p19: hidden frame]
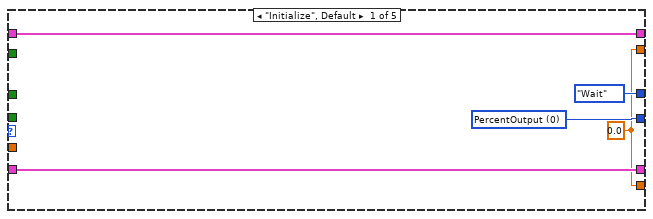
[diagram p20: hidden frame]
diagram:
  # "Pneumatics Controls"
  # "PressureSensor"
  # "Vn=V0/(.004*p0+.1)\n\np0 know pressure 120psi\nVo sensor output 2.8V\nVn normalized Replace Vsup 4.83V"
  # "Hype Train"
  # "Match/Robot Info"
  # "DB/Stings\n5)Gyro\n6)ShootVelocity\n7)TDistance\n8)Adjustment\n9)AutoState"
  # "DB/Stings\n0)Pressure\n1)LeftEnc\n2)RightEnc\n3)Tx\n4)TxSet"
  # "Joystick 2\nLeftx2: Manual Turret\nLefty2\nLeftTrigger2: TrackTarget\nRightTrigger2: KickUp Ball\nRightX2:\nRightY2:\n\nX2: Center Turret\nCircle2: Reverse Intake\nSquare2: Track No AutoSpin\nTriangle2:\nLeftBumper2: High Shot Spin Up\nRightBumper2: Low Shot Spin Up\nShare2: BackStep Climb\nOption2: AdvanceStep Climb\n\nPOV2: Adjust Distance & TxSet"
  # "Joystick 1\nLeftx1: Steering Drive\nLefty1:\nLeftTrigger1: Reverse Drive\nRightTrigger1: Forward Drive\nRightX1:\nRightY1:\n\nX1: Toggle Intake\nCircle1: Reverse Intake\nSquare1: Toggle Conveyor\nTriangle1:\nLeftBumper1: Slow Reverse Drive\nRightBumper1: Slow Forward Drive\nShare1: Compressor Toggle\nOption1:\n\nPOV1: Control Turn & SuperSlow"
  # "Enc: Inches/Count\nCircumference/CPR/GB Ratio\n4*Pi/2048/7.56"
  # "2048cpr with 4inch wheels"
  # "GyroSensors"
  # "DriveENC"
  # "stream\n0:SidebySide\n1:PiP Lime(usb)\n2:PiP USB(lime)"
  # "camMode\n0:Vision\n1:Basic"
  # "ledMode\n0: Pipeline\n1:Off\n2:Blink\n3:On"
  # "Shoot:\nAutoShot(w/Dist): LeftTrigger2\nHighShot(static): LeftBumper2\nLowShot(static): RightBumper2\nAdjust SpeedSets: POV1 0 & 180"
  # "Shooter Controls"
  # "Turret:\nManual: LeftX2\nPID: LeftTrigger2\nAutoCenter: X2\nTxAdjust: POV2 90 & 270"
  # "Turret Controls"
  # "Conveyor: Square1 (Toggle)\n                   X1 Or RightTrigger2 \n                  (Override Wait->ON)\nEject: Circle1 OR Circle2"
  # "Conveyor Controls"
  # "KickUp: RightTrigger2\nEject: Circle1 OR Circle2"
  # "Intake: X1\nEject: Circle1 OR Circle2"
  # "Forward: RightTrigger1\nReverse: LeftTrigger1\nSlowForward: RightBumper1\nSlowReverse: LeftBumper1"
  # "KickUp Controls"
  # "Limelight Data"
  # "Intake Controls"
  # "DriveTrain Controls"
  n1 = call <vilib>:"CTRE_Phoenix_MotorControl_RefNumRegistryGet.vi"("refnum name"="Right1") -> ("PhoenixMotorControlDevRef"=w1:T20)  [unwired: 9 in, 1 out]
  n2 = call <vilib>:"CTRE_Phoenix_MotorControl_RefNumRegistryGet.vi"("refnum name"="Right2") -> ("PhoenixMotorControlDevRef"=w2:T20)  [unwired: 9 in, 1 out]
  n3 = call <vilib>:"CTRE_Phoenix_MotorControl_RefNumRegistryGet.vi"("refnum name"="Left2") -> ("PhoenixMotorControlDevRef"=w3:T20)  [unwired: 9 in, 1 out]
  n4 = call <vilib>:"CTRE_Phoenix_MotorControl_RefNumRegistryGet.vi"("refnum name"="Left1") -> ("PhoenixMotorControlDevRef"=w4:T20)  [unwired: 9 in, 1 out]
  n5 = call <vilib>:"CTRE_Phoenix_MotorControl_RefNumRegistryGet.vi"("refnum name"="Shoot2") -> ("PhoenixMotorControlDevRef"=w10:T20)  [unwired: 9 in, 1 out]
  n6 = call <vilib>:"CTRE_Phoenix_MotorControl_RefNumRegistryGet.vi"("refnum name"="Shoot") -> ("PhoenixMotorControlDevRef"=w9:T20)  [unwired: 9 in, 1 out]
  n7 = while {
    tunnel: w10 -> [w75]
    tunnel: w9 -> [w68]
    tunnel: w4 -> [w67]
    tunnel: w3 -> [w64]
    tunnel: w2 -> [w63]
    tunnel: w1 -> [w60]
    stop <- w56 stop-if-true
    n8 = Wait (ms)(milliseconds to wait=u32 10) -> ()  [unwired: 1 out]
    n9 = call-poly <vilib>:"CTRE_Phoenix_MotorController_Get_TalonFX.vi"("PhoenixMotorControlDevRef"=w75) -> ("PhoenixMotorControlDevRef"=w76:T20, "Has Reset Occurred?"=w78:bool)  [unwired: 9 in, 4 out]
    n10 = call-poly <vilib>:"CTRE_Phoenix_MotorController_Get_TalonFX.vi"("PhoenixMotorControlDevRef"=w68) -> ("PhoenixMotorControlDevRef"=w73:T20, "Has Reset Occurred?"=w72:bool)  [unwired: 9 in, 4 out]
    n11 = call-poly <vilib>:"CTRE_Phoenix_MotorController_Get_TalonFX.vi"("PhoenixMotorControlDevRef"=w60) -> ("PhoenixMotorControlDevRef"=w58:T20, "Has Reset Occurred?"=w59:bool)  [unwired: 9 in, 4 out]
    n12 = call-poly <vilib>:"CTRE_Phoenix_MotorController_Get_TalonFX.vi"("PhoenixMotorControlDevRef"=w63) -> ("PhoenixMotorControlDevRef"=w61:T20, "Has Reset Occurred?"=w62:bool)  [unwired: 9 in, 4 out]
    n13 = call-poly <vilib>:"CTRE_Phoenix_MotorController_Get_TalonFX.vi"("PhoenixMotorControlDevRef"=w64) -> ("PhoenixMotorControlDevRef"=w65:T20, "Has Reset Occurred?"=w66:bool)  [unwired: 9 in, 4 out]
    n14 = call-poly <vilib>:"CTRE_Phoenix_MotorController_Get_TalonFX.vi"("PhoenixMotorControlDevRef"=w67) -> ("PhoenixMotorControlDevRef"=w70:T20, "Has Reset Occurred?"=w71:bool)  [unwired: 9 in, 4 out]
    n15 = case shown="True" w78 {
      tunnel: "ShootConfig2" -> [_ w149]
      tunnel: w76 -> [_ w148]
      frame False {
      }
      frame True {
        w142 = T8 1 items=["Integrated Sensor"=1, "Sensor Sum (S0 + S1)"=9, "Sensor Difference (D0 - D1)"=10, "Remote Source 0"=11, "Remote Source 1"=12, "None"=14, "Software Emulated"=15] ("Talon FX Feedback Device")
        n16 = call <vilib>:"CTRE_Phoenix_MotorControl_ConfigAllSettings_TalonFX.vi"("Talon FX Configurables"=w149, "PhoenixMotorControlDevRef"=w148) -> ("PhoenixMotorControlDevRef"=w140:T20)  [unwired: 8 in, 1 out]
        n17 = call <vilib>:"CTRE_Phoenix_MotorControl_SetInverted_TalonFX.vi"("Invert Type"=CTRE_Phoenix_MotorControl_TalonFXInvertType."Clockwise", "PhoenixMotorControlDevRef"=w140) -> ("error out"=w146:errorcluster, "PhoenixMotorControlDevRef"=w145:T20)  [unwired: 8 in]
        n18 = call <vilib>:"CTRE_Phoenix_MotorControl_SetNeutralMode.vi"("error in (no error)"=w146, "Motor Control Neutral Mode"=CTRE_Phoenix_MotorControl_NeutralMode."Override to Coast", "PhoenixMotorControlDevRef"=w145) -> ("error out"=w147:errorcluster, "PhoenixMotorControlDevRef"=w141:T20)  [unwired: 7 in]
        n19 = call <vilib>:"CTRE_Phoenix_MotorControl_ConfigSelectedFeedbackSensor_TalonFX.vi"("error in (no error)"=w147, "Talon FX Feedback Device"=w142, "PhoenixMotorControlDevRef"=w141) -> ()  [unwired: 7 in, 2 out]
      }
    }
    n20 = case shown="True" w72 {
      tunnel: "ShootConfig1" -> [_ w139]
      tunnel: w73 -> [_ w138]
      frame False {
      }
      frame True {
        w136 = T8 1 items=["Integrated Sensor"=1, "Sensor Sum (S0 + S1)"=9, "Sensor Difference (D0 - D1)"=10, "Remote Source 0"=11, "Remote Source 1"=12, "None"=14, "Software Emulated"=15] ("Talon FX Feedback Device")
        n21 = call <vilib>:"CTRE_Phoenix_MotorControl_ConfigAllSettings_TalonFX.vi"("Talon FX Configurables"=w139, "PhoenixMotorControlDevRef"=w138) -> ("PhoenixMotorControlDevRef"=w130:T20)  [unwired: 8 in, 1 out]
        n22 = call <vilib>:"CTRE_Phoenix_MotorControl_SetInverted_TalonFX.vi"("Invert Type"=CTRE_Phoenix_MotorControl_TalonFXInvertType."Counter-Clockwise", "PhoenixMotorControlDevRef"=w130) -> ("error out"=w132:errorcluster, "PhoenixMotorControlDevRef"=w133:T20)  [unwired: 8 in]
        n23 = call <vilib>:"CTRE_Phoenix_MotorControl_SetNeutralMode.vi"("error in (no error)"=w132, "Motor Control Neutral Mode"=CTRE_Phoenix_MotorControl_NeutralMode."Override to Coast", "PhoenixMotorControlDevRef"=w133) -> ("error out"=w131:errorcluster, "PhoenixMotorControlDevRef"=w137:T20)  [unwired: 7 in]
        n24 = call <vilib>:"CTRE_Phoenix_MotorControl_ConfigSelectedFeedbackSensor_TalonFX.vi"("error in (no error)"=w131, "Talon FX Feedback Device"=w136, "PhoenixMotorControlDevRef"=w137) -> ()  [unwired: 7 in, 2 out]
      }
    }
    n25 = case shown="True" w59 {
      tunnel: w58 -> [_ w81]
      tunnel: "DriveConfig" -> [_ w79]
      frame False {
      }
      frame True {
        w89 = T8 1 items=["Integrated Sensor"=1, "Sensor Sum (S0 + S1)"=9, "Sensor Difference (D0 - D1)"=10, "Remote Source 0"=11, "Remote Source 1"=12, "None"=14, "Software Emulated"=15] ("Talon FX Feedback Device")
        n26 = call <vilib>:"CTRE_Phoenix_MotorControl_ConfigAllSettings_TalonFX.vi"("Talon FX Configurables"=w79, "PhoenixMotorControlDevRef"=w81) -> ("PhoenixMotorControlDevRef"=w80:T20)  [unwired: 8 in, 1 out]
        n27 = call <vilib>:"CTRE_Phoenix_MotorControl_SetInverted_TalonFX.vi"("Invert Type"=CTRE_Phoenix_MotorControl_TalonFXInvertType."Clockwise", "PhoenixMotorControlDevRef"=w80) -> ("PhoenixMotorControlDevRef"=w86:T20)  [unwired: 8 in, 1 out]
        n28 = call <vilib>:"CTRE_Phoenix_MotorControl_SetNeutralMode.vi"("Motor Control Neutral Mode"=CTRE_Phoenix_MotorControl_NeutralMode."Override to Brake", "PhoenixMotorControlDevRef"=w86) -> ("error out"=w85:errorcluster, "PhoenixMotorControlDevRef"=w90:T20)  [unwired: 8 in]
        n29 = call <vilib>:"CTRE_Phoenix_MotorControl_ConfigSelectedFeedbackSensor_TalonFX.vi"("error in (no error)"=w85, "Talon FX Feedback Device"=w89, "PhoenixMotorControlDevRef"=w90) -> ("error out"=w82:errorcluster, "PhoenixMotorControlDevRef"=w83:T20)  [unwired: 7 in]
        n30 = call <vilib>:"CTRE_Phoenix_MotorControl_ConfigSensorInitializationStrategy.vi"("error in (no error)"=w82, "Sensor Initialization Strategy"=CTRE_Phoenix_CANcoder_SensorInitializationStrategy."Boot To Zero", "PhoenixMotorControlDevRef"=w83) -> ()  [unwired: 7 in, 2 out]
      }
    }
    n31 = case shown="True" w62 {
      tunnel: w61 -> [_ w92]
      tunnel: "DriveConfig" -> [_ w93]
      frame False {
      }
      frame True {
        w95 = T8 1 items=["Integrated Sensor"=1, "Sensor Sum (S0 + S1)"=9, "Sensor Difference (D0 - D1)"=10, "Remote Source 0"=11, "Remote Source 1"=12, "None"=14, "Software Emulated"=15] ("Talon FX Feedback Device")
        n32 = call <vilib>:"CTRE_Phoenix_MotorControl_ConfigAllSettings_TalonFX.vi"("Talon FX Configurables"=w93, "PhoenixMotorControlDevRef"=w92) -> ("PhoenixMotorControlDevRef"=w91:T20)  [unwired: 8 in, 1 out]
        n33 = call <vilib>:"CTRE_Phoenix_MotorControl_SetInverted_TalonFX.vi"("Invert Type"=CTRE_Phoenix_MotorControl_TalonFXInvertType."Clockwise", "PhoenixMotorControlDevRef"=w91) -> ("error out"=w100:errorcluster, "PhoenixMotorControlDevRef"=w99:T20)  [unwired: 8 in]
        n34 = call <vilib>:"CTRE_Phoenix_MotorControl_SetNeutralMode.vi"("error in (no error)"=w100, "Motor Control Neutral Mode"=CTRE_Phoenix_MotorControl_NeutralMode."Override to Coast", "PhoenixMotorControlDevRef"=w99) -> ("error out"=w101:errorcluster, "PhoenixMotorControlDevRef"=w98:T20)  [unwired: 7 in]
        n35 = call <vilib>:"CTRE_Phoenix_MotorControl_ConfigSelectedFeedbackSensor_TalonFX.vi"("error in (no error)"=w101, "Talon FX Feedback Device"=w95, "PhoenixMotorControlDevRef"=w98) -> ("error out"=w103:errorcluster, "PhoenixMotorControlDevRef"=w102:T20)  [unwired: 7 in]
        n36 = call <vilib>:"CTRE_Phoenix_MotorControl_ConfigSensorInitializationStrategy.vi"("error in (no error)"=w103, "Sensor Initialization Strategy"=CTRE_Phoenix_CANcoder_SensorInitializationStrategy."Boot To Zero", "PhoenixMotorControlDevRef"=w102) -> ()  [unwired: 7 in, 2 out]
      }
    }
    n37 = case shown="True" w66 {
      tunnel: "DriveConfig" -> [_ w116]
      tunnel: w65 -> [_ w115]
      frame False {
      }
      frame True {
        w111 = T8 1 items=["Integrated Sensor"=1, "Sensor Sum (S0 + S1)"=9, "Sensor Difference (D0 - D1)"=10, "Remote Source 0"=11, "Remote Source 1"=12, "None"=14, "Software Emulated"=15] ("Talon FX Feedback Device")
        n38 = call <vilib>:"CTRE_Phoenix_MotorControl_ConfigAllSettings_TalonFX.vi"("Talon FX Configurables"=w116, "PhoenixMotorControlDevRef"=w115) -> ("PhoenixMotorControlDevRef"=w104:T20)  [unwired: 8 in, 1 out]
        n39 = call <vilib>:"CTRE_Phoenix_MotorControl_SetInverted_TalonFX.vi"("Invert Type"=CTRE_Phoenix_MotorControl_TalonFXInvertType."Counter-Clockwise", "PhoenixMotorControlDevRef"=w104) -> ("error out"=w109:errorcluster, "PhoenixMotorControlDevRef"=w114:T20)  [unwired: 8 in]
        n40 = call <vilib>:"CTRE_Phoenix_MotorControl_SetNeutralMode.vi"("error in (no error)"=w109, "Motor Control Neutral Mode"=CTRE_Phoenix_MotorControl_NeutralMode."Override to Coast", "PhoenixMotorControlDevRef"=w114) -> ("error out"=w108:errorcluster, "PhoenixMotorControlDevRef"=w110:T20)  [unwired: 7 in]
        n41 = call <vilib>:"CTRE_Phoenix_MotorControl_ConfigSelectedFeedbackSensor_TalonFX.vi"("error in (no error)"=w108, "Talon FX Feedback Device"=w111, "PhoenixMotorControlDevRef"=w110) -> ("error out"=w105:errorcluster, "PhoenixMotorControlDevRef"=w106:T20)  [unwired: 7 in]
        n42 = call <vilib>:"CTRE_Phoenix_MotorControl_ConfigSensorInitializationStrategy.vi"("error in (no error)"=w105, "Sensor Initialization Strategy"=CTRE_Phoenix_CANcoder_SensorInitializationStrategy."Boot To Zero", "PhoenixMotorControlDevRef"=w106) -> ()  [unwired: 7 in, 2 out]
      }
    }
    n43 = case shown="True" w71 {
      tunnel: "DriveConfig" -> [_ w129]
      tunnel: w70 -> [_ w128]
      frame False {
      }
      frame True {
        w124 = T8 1 items=["Integrated Sensor"=1, "Sensor Sum (S0 + S1)"=9, "Sensor Difference (D0 - D1)"=10, "Remote Source 0"=11, "Remote Source 1"=12, "None"=14, "Software Emulated"=15] ("Talon FX Feedback Device")
        n44 = call <vilib>:"CTRE_Phoenix_MotorControl_ConfigAllSettings_TalonFX.vi"("Talon FX Configurables"=w129, "PhoenixMotorControlDevRef"=w128) -> ("PhoenixMotorControlDevRef"=w117:T20)  [unwired: 8 in, 1 out]
        n45 = call <vilib>:"CTRE_Phoenix_MotorControl_SetInverted_TalonFX.vi"("Invert Type"=CTRE_Phoenix_MotorControl_TalonFXInvertType."Counter-Clockwise", "PhoenixMotorControlDevRef"=w117) -> ("error out"=w122:errorcluster, "PhoenixMotorControlDevRef"=w127:T20)  [unwired: 8 in]
        n46 = call <vilib>:"CTRE_Phoenix_MotorControl_SetNeutralMode.vi"("error in (no error)"=w122, "Motor Control Neutral Mode"=CTRE_Phoenix_MotorControl_NeutralMode."Override to Brake", "PhoenixMotorControlDevRef"=w127) -> ("error out"=w121:errorcluster, "PhoenixMotorControlDevRef"=w123:T20)  [unwired: 7 in]
        n47 = call <vilib>:"CTRE_Phoenix_MotorControl_ConfigSelectedFeedbackSensor_TalonFX.vi"("error in (no error)"=w121, "Talon FX Feedback Device"=w124, "PhoenixMotorControlDevRef"=w123) -> ("error out"=w118:errorcluster, "PhoenixMotorControlDevRef"=w119:T20)  [unwired: 7 in]
        n48 = call <vilib>:"CTRE_Phoenix_MotorControl_ConfigSensorInitializationStrategy.vi"("error in (no error)"=w118, "Sensor Initialization Strategy"=CTRE_Phoenix_CANcoder_SensorInitializationStrategy."Boot To Zero", "PhoenixMotorControlDevRef"=w119) -> ()  [unwired: 7 in, 2 out]
      }
    }
    n49 = call "Elapsed Time3"() -> ("Time has Elapsed"=w56:bool)  [unwired: 12 in, 7 out]
  }
  n50 = while {
    tunnel: w9 -> [w199]
    shift-right: [w196] -> _
    shift-left: T17."Initialize" -> [w197]
    shift-right: [w175] -> _
    shift-left: -5.0 ("x") -> [w172]
    tunnel: w10 -> [w169]
    stop <- FALSE stop-if-true
    n51 = global read "Robot Global Data.vi" "POV2"() -> (w184:i16)
    n52 = global read "Robot Global Data.vi" "RightBumper2"() -> (w191:bool)
    n53 = call-poly <vilib>:"CTRE_Phoenix_MotorController_Get_TalonFX.vi"("PhoenixMotorControlDevRef"=w199) -> ("PhoenixMotorControlDevRef"=w188:T20, "Velocity (Raw Sensor Units per 100 ms)"=w187:i32)  [unwired: 11 in, 2 out]
    n54 = global read "Robot Global Data.vi" "LeftBumper2"() -> (w192:bool)
    n55 = global write "Robot Global Data.vi" "ShooterVel"(w187) -> ()
    n56 = global read "Robot Global Data.vi" "RightTrigger2"() -> (w162:dbl)
    n57 = Equal?(x=i16 0 ("POV1"), y=w184) -> (x = y?=w183:bool)
    n58 = Equal?(x=w184, y=i16 180 ("POV1")) -> (x = y?=w182:bool)
    n59 = global read "Robot Global Data.vi" "TDistance"() -> (w160:dbl)
    n60 = call-poly <vilib>:"CTRE_Phoenix_MotorController_Get_TalonFX.vi"("PhoenixMotorControlDevRef"=w169) -> ("PhoenixMotorControlDevRef"=w166:T20, "Velocity (Raw Sensor Units per 100 ms)"=w168:i32)  [unwired: 11 in, 2 out]
    n61 = global write "Robot Global Data.vi" "ShooterVel2"(w168) -> ()
    n62 = call <vilib>:"Edge Detector.vi"("Mode"=enum16{"Rising", "Falling", "Any"}."Rising", "Input"=w183) -> ("Output"=w181:bool)  [unwired: 9 in]
    n63 = call <vilib>:"Edge Detector.vi"("Mode"=enum16{"Rising", "Falling", "Any"}."Rising", "Input"=w182) -> ("Output"=w180:bool)  [unwired: 9 in]
    n64 = Greater?(x=w162, y=0.2 ("x")) -> (0:w157:bool)
    n65 = global read "Robot Global Data.vi" "LeftTrigger2"() -> (w194:dbl)
    n66 = Select(t=5.0, s=w181, f=0.0) -> (s? t:f=w177:dbl)
    n67 = Select(t=-5.0, s=w180, f=0.0) -> (s? t:f=w176:dbl)
    n68 = global read "Robot Global Data.vi" "Triangle2"() -> (w150:bool)
    n69 = feedback #1() -> (w159:dbl)  [unwired: 1 in]
    n70 = call <vilib>:"Edge Detector.vi"("Mode"=enum16{"Rising", "Falling", "Any"}."Rising", "Input"=w157) -> ("Output"=w156:bool)  [unwired: 9 in]
    n71 = Select(t=w159, s=w157, f=w160) -> (s? t:f=w153:dbl)
    n72 = Greater?(x=w194, y=0.25 ("x")) -> (0:w193:bool)
    n73 = Compound Arithmetic op=ADD(w177, w176, w172) -> (w175:dbl)
    n74 = Or(x=w193, y=w150) -> (x .or. y?=w151:bool)
    n75 = Subtract(x=w153, y=10.0) -> (x-y=w154:dbl)
    n76 = Select(t=w154, s=w156, f=w153) -> (s? t:f=w155:dbl)
    n77 = feedback-in #1(w155) -> ()
    n78 = case shown="\"AutoShot\"" w197 {
      selector: w197 -> [_ w217 w227 w235 w247]
      tunnel: [w204 w218 w228 w239 w251] -> w198
      tunnel: w188 -> [w204 w218 w228 w239 w251]
      tunnel: [w200 w206 3000.0 ("Output") 5500.0 ("Result") w242] -> w164
      tunnel: [T17."Wait" w205 w221 w237 w249] -> w196
      tunnel: w151 -> [_ w211 w220 _ w248]
      tunnel: w192 -> [_ w210 _ w236 _]
      tunnel: w191 -> [_ w209 w229 _ _]
      tunnel: w153 -> [_ _ _ _ w244]
      tunnel: w175 -> [_ _ _ _ w240]
      tunnel: w166 -> [w202 w208 w226 w234 w246]
      tunnel: [w202 w208 w226 w234 w246] -> w167
      tunnel: [w201 w207 w225 w233 w245] -> w163
      tunnel: [w200 w206 3500.0 ("Output") 8000.0 ("Result") w243] -> w165
      frame "Initialize", Default {
        w200 = 0.0 ("Output")
        w201 = T27 0 items=["PercentOutput"=0, "Position"=1, "Velocity"=2, "Current"=3, "Follower"=5, "MotionProfile"=6, "MotionMagic"=7, "MotionProfileArc"=10, "Disabled"=15] ("Control Mode")
      }
      frame "Wait" {
        w206 = 0.0 ("Output")
        w207 = T27 0 items=["PercentOutput"=0, "Position"=1, "Velocity"=2, "Current"=3, "Follower"=5, "MotionProfile"=6, "MotionMagic"=7, "MotionProfileArc"=10, "Disabled"=15] ("Control Mode")
        n79 = Select(t=T17."LowShot", s=w209, f=w217) -> (s? t:f=w216:T17)
        n80 = Select(t=T17."HighShot", s=w210, f=w216) -> (s? t:f=w215:T17)
        n81 = Select(t=T17."AutoShot", s=w211, f=w215) -> (s? t:f=w205:T17)
      }
      frame "LowShot" {
        w225 = T27 2 items=["PercentOutput"=0, "Position"=1, "Velocity"=2, "Current"=3, "Follower"=5, "MotionProfile"=6, "MotionMagic"=7, "MotionProfileArc"=10, "Disabled"=15] ("Control Mode")
        # "4000"
        # "3500"
        n82 = Select(t=w227, s=w229, f=T17."Wait") -> (s? t:f=w222:T17)
        n83 = Select(t=T17."AutoShot", s=w220, f=w222) -> (s? t:f=w221:T17)
      }
      frame "HighShot" {
        w233 = T27 2 items=["PercentOutput"=0, "Position"=1, "Velocity"=2, "Current"=3, "Follower"=5, "MotionProfile"=6, "MotionMagic"=7, "MotionProfileArc"=10, "Disabled"=15] ("Control Mode")
        # "12000"
        # "8500"
        n84 = Select(t=w235, s=w236, f=T17."Wait") -> (s? t:f=w237:T17)
      }
      frame "AutoShot" {
        w245 = T27 2 items=["PercentOutput"=0, "Position"=1, "Velocity"=2, "Current"=3, "Follower"=5, "MotionProfile"=6, "MotionMagic"=7, "MotionProfileArc"=10, "Disabled"=15] ("Control Mode")
        n85 = Add(x=w244, y=w240) -> (x+y=w241:dbl)
        n86 = xnode "TopEq"("Td"=w241) -> ("Result"=w243:dbl)  [unwired: 1 in, 1 out]
        n87 = Select(t=w247, s=w248, f=T17."Wait") -> (s? t:f=w249:T17)
        n88 = xnode "BottomEq"("Td"=w241) -> ("Result"=w242:dbl)  [unwired: 1 in, 1 out]
      }
    }
    n89 = global write "Robot Global Data.vi" "Adjustment"(w175) -> ()
    n90 = Wait (ms)(milliseconds to wait=u32 20) -> ()  [unwired: 1 out]
    n91 = call <vilib>:"CTRE_Phoenix_MotorControl_Set.vi"("Output"=w164, "Control Mode"=w163, "PhoenixMotorControlDevRef"=w198) -> ()  [unwired: 7 in, 2 out]
    n92 = call <vilib>:"CTRE_Phoenix_MotorControl_Set.vi"("Output"=w165, "Control Mode"=w163, "PhoenixMotorControlDevRef"=w167) -> ()  [unwired: 7 in, 2 out]
  }
  n93 = call <vilib>:"WPI_MotorControlRefNum Registry Get.vi"("refnum name"="Turret") -> ("MotorControlDevRef"=w31:T20)  [unwired: 9 in, 1 out]
  n94 = call <vilib>:"Spark MAX Set Soft Limit Config.vi"("Soft Limit (0)"=-70.0, "Soft Limit Switch"=Spark_MAX_Limit_Direction."Reverse Limit", "MotorControlDeviceRef in"=w31) -> ("MotorControlDeviceRef out"=w34:T20)  [unwired: 7 in, 1 out]
  n95 = call <vilib>:"WPI_MotorControlRefNum Registry Get.vi"("refnum name"="Intake") -> ("MotorControlDevRef"=w54:T20)  [unwired: 9 in, 1 out]
  n96 = call <vilib>:"WPI_MotorControlRefNum Registry Get.vi"("refnum name"="KickUp") -> ("MotorControlDevRef"=w49:T20)  [unwired: 9 in, 1 out]
  n97 = call <vilib>:"WPI_MotorControlRefNum Registry Get.vi"("refnum name"="Conveyor") -> ("MotorControlDevRef"=w46:T20)  [unwired: 9 in, 1 out]
  n98 = call <vilib>:"Spark MAX Set Soft Limit Config.vi"("Soft Limit (0)"=90.0, "Soft Limit Switch"=Spark_MAX_Limit_Direction."Forward Limit", "MotorControlDeviceRef in"=w34) -> ("MotorControlDeviceRef out"=w28:T20)  [unwired: 7 in, 1 out]
  n99 = call <vilib>:"WPI_SolenoidRefNum Registry Get.vi"("refnum name"="FlipUp") -> ("SolenoidDevRef"=w12:T28)  [unwired: 9 in, 1 out]
  n100 = call <vilib>:"WPI_SolenoidRefNum Registry Get.vi"("refnum name"="Lift") -> ("SolenoidDevRef"=w13:T28)  [unwired: 9 in, 1 out]
  n101 = call <vilib>:"WPI_RobotDriveRefNum Registry Get.vi"("refnum name"="Drive") -> ("RobotDriveDevRef"=w52:T30)  [unwired: 1 in, 9 out]
  n102 = while {
    tunnel: w13 -> [w281]
    tunnel: w12 -> [w280]
    shift-right: [w277] -> _
    shift-left: T16."Initialize" -> [w272]
    stop <- FALSE stop-if-true
    n103 = global read "Robot Global Data.vi" "Option2"() -> (w276:bool)
    n104 = global read "Robot Global Data.vi" "Share2"() -> (w271:bool)
    n105 = call <vilib>:"Edge Detector.vi"("Mode"=enum16{"Rising", "Falling", "Any"}."Rising", "Input"=w271) -> ("Output"=w270:bool)  [unwired: 9 in]
    n106 = call <vilib>:"Edge Detector.vi"("Mode"=enum16{"Rising", "Falling", "Any"}."Rising", "Input"=w276) -> ("Output"=w275:bool)  [unwired: 9 in]
    n107 = case shown="\"UnClimb\"" w272 {
      selector: w272 -> [_ w286 w297 w310 w318 w325]
      tunnel: [WPI_SolenoidValue."Off" ("Value") WPI_SolenoidValue."Off" ("Value") WPI_SolenoidValue."On" ("Value") WPI_SolenoidValue."Off" ("Value") WPI_SolenoidValue."Off" ("Value") WPI_SolenoidValue."On" ("Value")] -> w279
      tunnel: [WPI_SolenoidValue."Off" ("Value") WPI_SolenoidValue."Off" ("Value") WPI_SolenoidValue."On" ("Value") WPI_SolenoidValue."On" ("Value") WPI_SolenoidValue."Off" ("Value") WPI_SolenoidValue."Off" ("Value")] -> w278
      tunnel: [T16."Wait" w287 w294 w305 w314 w326] -> w277
      tunnel: w275 -> [_ w288 w298 w307 w317 _]
      tunnel: w270 -> [_ _ w296 w304 w316 _]
      frame "Initialize", Default {
      }
      frame "Wait" {
        n108 = Select(t=T16."Extend", s=w288, f=w286) -> (s? t:f=w287:T16)
      }
      frame "Extend" {
        n109 = Select(t=T16."Midbar", s=w298, f=w297) -> (s? t:f=w295:T16)
        n110 = global write "Robot Global Data.vi" "AutoState"("Extend" ("AutoState")) -> ()
        n111 = Select(t=T16."Wait", s=w296, f=w295) -> (s? t:f=w294:T16)
      }
      frame "Midbar" {
        n112 = Select(t=T16."FlipOn", s=w307, f=w310) -> (s? t:f=w306:T16)
        n113 = global write "Robot Global Data.vi" "AutoState"("Midbar" ("AutoState")) -> ()
        n114 = Select(t=T16."Extend", s=w304, f=w306) -> (s? t:f=w305:T16)
      }
      frame "FlipOn" {
        n115 = Select(t=T16."UnClimb", s=w317, f=w318) -> (s? t:f=w315:T16)
        n116 = global write "Robot Global Data.vi" "AutoState"("FlipOn" ("AutoState")) -> ()
        n117 = Select(t=T16."Midbar", s=w316, f=w315) -> (s? t:f=w314:T16)
      }
      frame "UnClimb" {
        n118 = call "Elapsed Time2"("Time Target (s)"=0.5) -> ("Time has Elapsed"=w323:bool)  [unwired: 11 in, 7 out]
        n119 = global write "Robot Global Data.vi" "AutoState"("UnClimb" ("AutoState")) -> ()
        n120 = Select(t=T16."Wait", s=w323, f=w325) -> (s? t:f=w326:T16)
      }
    }
    n121 = Wait (ms)(milliseconds to wait=u32 30) -> ()  [unwired: 1 out]
    n122 = call-poly <vilib>:"WPI_SolenoidSet.vi"("Value"=w279, "SolenoidDevRef"=w281) -> ()  [unwired: 8 in, 2 out]
    n123 = call-poly <vilib>:"WPI_SolenoidSet.vi"("Value"=w278, "SolenoidDevRef"=w280) -> ()  [unwired: 8 in, 2 out]
  }
  n124 = while {
    shift-right: [w363] -> _
    shift-left: T19."Initialize" -> [w365]
    tunnel: w28 -> [w355]
    shift-right: [w333] -> _
    shift-left: 0.0 -> [w352]
    stop <- FALSE stop-if-true
    n125 = global read "Robot Global Data.vi" "POV2"() -> (w347:i16)
    n126 = call <vilib>:"Spark MAX Get Sensor Position.vi"("MotorControlDevRef in"=w355) -> ("Sensor Position"=w353:dbl, "MotorControlDevRef out"=w354:T20)  [unwired: 7 in, 2 out]
    n127 = global write "Robot Global Data.vi" "TurretPos"(w353) -> ()
    n128 = Equal?(x=i16 90 ("POV1"), y=w347) -> (x = y?=w348:bool)
    n129 = Equal?(x=w347, y=i16 270 ("POV1")) -> (x = y?=w349:bool)
    n130 = global read "Robot Global Data.vi" "RightTrigger2"() -> (w331:dbl)
    n131 = call <vilib>:"Edge Detector.vi"("Mode"=enum16{"Rising", "Falling", "Any"}."Rising", "Input"=w348) -> ("Output"=w337:bool)  [unwired: 9 in]
    n132 = call <vilib>:"Edge Detector.vi"("Mode"=enum16{"Rising", "Falling", "Any"}."Rising", "Input"=w349) -> ("Output"=w350:bool)  [unwired: 9 in]
    n133 = Select(t=1.0, s=w337, f=0.0) -> (s? t:f=w339:dbl)
    n134 = Select(t=-1.0, s=w350, f=0.0) -> (s? t:f=w351:dbl)
    n135 = Compound Arithmetic op=ADD(w339, w352, w351) -> (w333:dbl)
    n136 = Greater?(x=w331, y=0.25 ("x")) -> (0:w329:bool)
    n137 = global read "Robot Global Data.vi" "TDistance"() -> (w334:dbl)
    n138 = global read "Robot Global Data.vi" "LeftTrigger2"() -> (w361:dbl)
    n139 = global read "Robot Global Data.vi" "X2"() -> (w358:bool)
    n140 = global read "Robot Global Data.vi" "Square2"() -> (w335:bool)
    n141 = global read "Robot Global Data.vi" "LeftX2"() -> (w362:dbl)
    n142 = global read "Robot Global Data.vi" "Tx"() -> (w357:dbl)
    n143 = global read "Robot Global Data.vi" "Tv"() -> (w356:dbl)
    n144 = Greater?(x=w361, y=0.25 ("x")) -> (0:w359:bool)
    n145 = Compound Arithmetic op=OR(w359, w335) -> (w336:bool)
    n146 = case shown="\"PID\"" w365 {
      selector: w365 -> [_ w379 w394 w411]
      tunnel: [w370 w372 w398 w407] -> w364
      tunnel: w354 -> [w370 w372 w398 w407]
      tunnel: [T19."Manual" w377 w401 w410] -> w363
      tunnel: w362 -> [_ w371 _ _]
      tunnel: [0.0 ("LeftX2") w371 w381 w402] -> w332
      tunnel: w336 -> [_ w374 w400 _]
      tunnel: w358 -> [_ w373 _ w408]
      tunnel: w357 -> [_ _ w396 _]
      tunnel: w356 -> [_ _ w395 _]
      tunnel: w353 -> [_ _ _ w403]
      tunnel: w333 -> [_ _ w386 _]
      tunnel: w334 -> [_ _ w388 _]
      tunnel: w329 -> [_ _ w382 _]
      frame "Initialize", Default {
      }
      frame "Manual" {
        n147 = Select(t=T19."PID", s=w374, f=w379) -> (s? t:f=w378:T19)
        n148 = Select(t=T19."AutoCenter", s=w373, f=w378) -> (s? t:f=w377:T19)
      }
      frame "PID" {
        n149 = Multiply(x=w396, y=w395) -> (x*y=w384:dbl)
        n150 = Less Or Equal?(x=w388, y=90.0) -> (x <= y?=w389:bool)
        n151 = Select(t=sgl 0.8 ("Rumble"), s=w389, f=sgl 0.0 ("Rumble")) -> (s? t:f=w391:sgl)
        n152 = global write "Robot Global Data.vi" "Rumble"(w391) -> ()
        n153 = Select(t=w394, s=w400, f=T19."Manual") -> (s? t:f=w401:T19)
        n154 = call-poly <vilib>:"PID.vi"("output range"=cluster{"output high":dbl, "output low":dbl} {"output high"=1.0, "output low"=-1.0}, "PID gains"=T32 {"proportional gain (Kp)"=0.06, "integral time (Ki)"=0.01, "derivative time (Kd)"=0.0}, "process variable"=w384, "setpoint"=w386) -> ("output"=w387:dbl)  [unwired: 6 in, 1 out]
        n155 = Negate(x=w387) -> (-x=w383:dbl)
        n156 = Select(t=0.0, s=w382, f=w383) -> (s? t:f=w381:dbl)
      }
      frame "AutoCenter" {
        n157 = Select(t=w411, s=w408, f=T19."Manual") -> (s? t:f=w410:T19)
        n158 = call-poly <vilib>:"PID.vi"("output range"=cluster{"output high":dbl, "output low":dbl} {"output high"=1.0, "output low"=-1.0}, "PID gains"=T32 {"proportional gain (Kp)"=0.06, "integral time (Ki)"=0.01, "derivative time (Kd)"=0.0}, "process variable"=w403, "setpoint"=10.0) -> ("output"=w402:dbl)  [unwired: 6 in, 1 out]
      }
    }
    n159 = global write "Robot Global Data.vi" "TxAdj"(w333) -> ()
    n160 = call <vilib>:"WPI_MotorControlSetOutput.vi"("Output"=w332, "MotorControlDevRef"=w364) -> ()  [unwired: 7 in, 3 out]
    n161 = Wait (ms)(milliseconds to wait=u32 20) -> ()  [unwired: 1 out]
  }
  n162 = while {
    tunnel: w52 -> [w448]
    stop <- FALSE stop-if-true
    n163 = global read "Robot Global Data.vi" "POV1"() -> (w435:i16)
    n164 = global read "Robot Global Data.vi" "LeftTrigger1"() -> (w442:dbl)
    n165 = global read "Robot Global Data.vi" "RightTrigger1"() -> (w441:dbl)
    n166 = global read "Robot Global Data.vi" "LeftX1"() -> (w438:dbl)
    n167 = Equal?(x=i16 270 ("POV1"), y=w435) -> (x = y?=w436:bool)
    n168 = Equal?(x=w435, y=i16 90 ("POV1")) -> (x = y?=w437:bool)
    n169 = Negate(x=w442) -> (-x=w440:dbl)
    n170 = global read "Robot Global Data.vi" "POV1"() -> (w427:i16)
    n171 = Add(x=w440, y=w441) -> (x+y=w421:dbl)
    n172 = Select(t=-0.55, s=w437, f=w438) -> (s? t:f=w439:dbl)
    n173 = Select(t=0.55, s=w436, f=w439) -> (s? t:f=w414:dbl)
    n174 = Equal?(x=i16 0 ("POV1"), y=w427) -> (x = y?=w428:bool)
    n175 = Equal?(x=w427, y=i16 180 ("POV1")) -> (x = y?=w429:bool)
    n176 = global read "Robot Global Data.vi" "LeftBumper1"() -> (w447:bool)
    n177 = Select(t=-0.3, s=w429, f=w421) -> (s? t:f=w430:dbl)
    n178 = global read "Robot Global Data.vi" "RightBumper1"() -> (w446:bool)
    n179 = Select(t=0.3, s=w428, f=w430) -> (s? t:f=w422:dbl)
    n180 = global read "Robot Global Data.vi" "RightTrigger2"() -> (w417:dbl)
    n181 = Select(t=-0.55, s=w447, f=w422) -> (s? t:f=w445:dbl)
    n182 = Select(t=0.55, s=w446, f=w445) -> (s? t:f=w420:dbl)
    n183 = Greater?(x=w417, y=0.2) -> (0:w413:bool)
    n184 = Select(t=0.0, s=w413, f=w420) -> (s? t:f=w419:dbl)
    n185 = Select(t=0.0, s=w413, f=w414) -> (s? t:f=w415:dbl)
    n186 = Wait (ms)(milliseconds to wait=u32 30) -> ()  [unwired: 1 out]
    n187 = call-poly <vilib>:"WPI_RobotDriveArcadeDrive.vi"("Y axis value"=w419, "X axis value"=w415, "RobotDriveDevRef"=w448) -> ()  [unwired: 6 in, 3 out]
  }
  n188 = while {
    tunnel: w49 -> [w460]
    shift-right: [w458] -> _
    shift-left: enum16{"Initialize", "Wait", "On", "Reverse"}."Initialize" -> [w459]
    stop <- FALSE stop-if-true
    n189 = global read "Robot Global Data.vi" "RightTrigger2"() -> (w454:dbl)
    n190 = global read "Robot Global Data.vi" "Circle1"() -> (w453:bool)
    n191 = global read "Robot Global Data.vi" "Circle2"() -> (w452:bool)
    n192 = Or(x=w452, y=w453) -> (x .or. y?=w451:bool)
    n193 = Greater?(x=w454, y=0.25 ("x")) -> (0:w456:bool)
    n194 = case shown="\"On\"" w459 {
      selector: w459 -> [_ w473 w479 w485]
      tunnel: [w466 w475 w477 w482] -> w461
      tunnel: w460 -> [w466 w475 w477 w482]
      tunnel: [enum16{"Initialize", "Wait", "On", "Reverse"}."Wait" w471 w480 w487] -> w458
      tunnel: [0.0 ("Output") 0.0 ("Output") 0.8 ("Output") -0.75 ("Output")] -> w457
      tunnel: w456 -> [_ w470 w481 _]
      tunnel: w451 -> [_ w468 _ w486]
      frame "Initialize", Default {
      }
      frame "Wait" {
        n195 = Select(t=enum16{"Initialize", "Wait", "On", "Reverse"}."On", s=w470, f=w473) -> (s? t:f=w472:enum16{"Initialize", "Wait", "On", "Reverse"})
        n196 = Select(t=enum16{"Initialize", "Wait", "On", "Reverse"}."Reverse", s=w468, f=w472) -> (s? t:f=w471:enum16{"Initialize", "Wait", "On", "Reverse"})
      }
      frame "On" {
        n197 = Select(t=w479, s=w481, f=enum16{"Initialize", "Wait", "On", "Reverse"}."Wait") -> (s? t:f=w480:enum16{"Initialize", "Wait", "On", "Reverse"})
      }
      frame "Reverse" {
        n198 = Select(t=w485, s=w486, f=enum16{"Initialize", "Wait", "On", "Reverse"}."Wait") -> (s? t:f=w487:enum16{"Initialize", "Wait", "On", "Reverse"})
      }
    }
    n199 = call <vilib>:"WPI_MotorControlSetOutput.vi"("Output"=w457, "MotorControlDevRef"=w461) -> ()  [unwired: 7 in, 3 out]
    n200 = Wait (ms)(milliseconds to wait=u32 30) -> ()  [unwired: 1 out]
  }
  n201 = while {
    tunnel: w54 -> [w498]
    shift-right: [w496] -> _
    shift-left: enum16{"Initialize", "Wait", "On", "Reverse"}."Initialize" -> [w497]
    stop <- FALSE stop-if-true
    n202 = global read "Robot Global Data.vi" "Circle1"() -> (w494:bool)
    n203 = global read "Robot Global Data.vi" "Circle2"() -> (w492:bool)
    n204 = global read "Robot Global Data.vi" "X1"() -> (w490:bool)
    n205 = Or(x=w492, y=w494) -> (x .or. y?=w493:bool)
    n206 = call <vilib>:"Edge Detector.vi"("Mode"=enum16{"Rising", "Falling", "Any"}."Rising", "Input"=w490) -> ("Output"=w489:bool)  [unwired: 9 in]
    n207 = case shown="\"On\"" w497 {
      selector: w497 -> [_ w513 w522 w530]
      tunnel: [w505 w515 w523 w527] -> w499
      tunnel: w498 -> [w505 w515 w523 w527]
      tunnel: [enum16{"Initialize", "Wait", "On", "Reverse"}."Wait" w511 w520 w532] -> w496
      tunnel: [0.0 ("Output") 0.0 ("Output") 0.8 ("Output") -0.75 ("Output")] -> w495
      tunnel: w489 -> [_ w510 w525 _]
      tunnel: w493 -> [_ w508 w517 w531]
      frame "Initialize", Default {
        n208 = global write "Robot Global Data.vi" "IntakeOn?"(FALSE ("IntakeOn?")) -> ()
      }
      frame "Wait" {
        n209 = Select(t=enum16{"Initialize", "Wait", "On", "Reverse"}."On", s=w510, f=w513) -> (s? t:f=w512:enum16{"Initialize", "Wait", "On", "Reverse"})
        n210 = Select(t=enum16{"Initialize", "Wait", "On", "Reverse"}."Reverse", s=w508, f=w512) -> (s? t:f=w511:enum16{"Initialize", "Wait", "On", "Reverse"})
        n211 = global write "Robot Global Data.vi" "IntakeOn?"(FALSE ("IntakeOn?")) -> ()
      }
      frame "On" {
        n212 = Select(t=enum16{"Initialize", "Wait", "On", "Reverse"}."Wait", s=w525, f=w522) -> (s? t:f=w519:enum16{"Initialize", "Wait", "On", "Reverse"})
        n213 = global write "Robot Global Data.vi" "IntakeOn?"(TRUE ("IntakeOn?")) -> ()
        n214 = Select(t=enum16{"Initialize", "Wait", "On", "Reverse"}."Reverse", s=w517, f=w519) -> (s? t:f=w520:enum16{"Initialize", "Wait", "On", "Reverse"})
      }
      frame "Reverse" {
        n215 = Select(t=w530, s=w531, f=enum16{"Initialize", "Wait", "On", "Reverse"}."Wait") -> (s? t:f=w532:enum16{"Initialize", "Wait", "On", "Reverse"})
        n216 = global write "Robot Global Data.vi" "IntakeOn?"(FALSE ("IntakeOn?")) -> ()
      }
    }
    n217 = Negate(x=w495) -> (-x=w488:dbl)
    n218 = call <vilib>:"WPI_MotorControlSetOutput.vi"("Output"=w488, "MotorControlDevRef"=w499) -> ()  [unwired: 7 in, 3 out]
    n219 = Wait (ms)(milliseconds to wait=u32 30) -> ()  [unwired: 1 out]
  }
  n220 = while {
    tunnel: w46 -> [w549]
    shift-right: [w547] -> _
    shift-left: enum16{"Initialize", "Wait", "On", "Reverse"}."Initialize" -> [w548]
    stop <- FALSE stop-if-true
    n221 = global read "Robot Global Data.vi" "IntakeOn?"() -> (w535:bool)
    n222 = global read "Robot Global Data.vi" "Square1"() -> (w545:bool)
    n223 = global read "Robot Global Data.vi" "RightTrigger2"() -> (w538:dbl)
    n224 = global read "Robot Global Data.vi" "Circle1"() -> (w543:bool)
    n225 = global read "Robot Global Data.vi" "Circle2"() -> (w542:bool)
    n226 = global read "Robot Global Data.vi" "X1"() -> (w534:bool)
    n227 = call <vilib>:"Edge Detector.vi"("Mode"=enum16{"Rising", "Falling", "Any"}."Rising", "Input"=w545) -> ("Output"=w540:bool)  [unwired: 9 in]
    n228 = Or(x=w542, y=w543) -> (x .or. y?=w541:bool)
    n229 = Greater?(x=w538, y=0.25 ("x")) -> (0:w537:bool)
    n230 = Compound Arithmetic op=OR(w537, w534, w535) -> (w536:bool)
    n231 = case shown="\"On\"" w548 {
      selector: w548 -> [_ w566 w573 w580]
      tunnel: [w555 w567 w575 w577] -> w550
      tunnel: w549 -> [w555 w567 w575 w577]
      tunnel: [enum16{"Initialize", "Wait", "On", "Reverse"}."Wait" w564 w570 w582] -> w547
      tunnel: [0.0 ("Output") w557 0.75 ("Output") -0.75 ("Output")] -> w546
      tunnel: w541 -> [_ w562 w568 w581]
      tunnel: w540 -> [_ w560 w574 _]
      tunnel: w536 -> [_ w559 _ _]
      frame "Initialize", Default {
      }
      frame "Wait" {
        n232 = Select(t=enum16{"Initialize", "Wait", "On", "Reverse"}."On", s=w560, f=w566) -> (s? t:f=w565:enum16{"Initialize", "Wait", "On", "Reverse"})
        n233 = Select(t=enum16{"Initialize", "Wait", "On", "Reverse"}."Reverse", s=w562, f=w565) -> (s? t:f=w564:enum16{"Initialize", "Wait", "On", "Reverse"})
        n234 = Select(t=0.85, s=w559, f=0.0 ("Output")) -> (s? t:f=w557:dbl)
      }
      frame "On" {
        n235 = Select(t=enum16{"Initialize", "Wait", "On", "Reverse"}."Wait", s=w574, f=w573) -> (s? t:f=w571:enum16{"Initialize", "Wait", "On", "Reverse"})
        n236 = Select(t=enum16{"Initialize", "Wait", "On", "Reverse"}."Reverse", s=w568, f=w571) -> (s? t:f=w570:enum16{"Initialize", "Wait", "On", "Reverse"})
      }
      frame "Reverse" {
        n237 = Select(t=w580, s=w581, f=enum16{"Initialize", "Wait", "On", "Reverse"}."Wait") -> (s? t:f=w582:enum16{"Initialize", "Wait", "On", "Reverse"})
      }
    }
    n238 = Negate(x=w546) -> (-x=w533:dbl)
    n239 = Wait (ms)(milliseconds to wait=u32 30) -> ()  [unwired: 1 out]
    n240 = call <vilib>:"WPI_MotorControlSetOutput.vi"("Output"=w533, "MotorControlDevRef"=w550) -> ()  [unwired: 7 in, 3 out]
  }
  n241 = disable-structure shown="Disabled" {
    frame Disabled {
      n242 = call <vilib>:"WPI_SolenoidRefNum Registry Get.vi"("refnum name"="Lift") -> ("SolenoidDevRef"=w587:T28)  [unwired: 9 in, 1 out]
      n243 = call <vilib>:"WPI_SolenoidRefNum Registry Get.vi"("refnum name"="FlipUp") -> ("SolenoidDevRef"=w584:T28)  [unwired: 9 in, 1 out]
      n244 = while {
        shift-right: [w602] -> _
        shift-left: enum16{"Initialize", "Off", "On"}."Initialize" -> [w606]
        tunnel: w587 -> [w605]
        shift-right: [w596] -> _
        shift-left: enum16{"Initialize", "Off", "On"}."Initialize" -> [w601]
        tunnel: w584 -> [w600]
        stop <- FALSE stop-if-true
        w592 = TRUE ("Reset")
        w595 = TRUE ("Reset")
        n245 = global read "Robot Global Data.vi" "Share2"() -> (w603:bool)
        n246 = global read "Robot Global Data.vi" "Option2"() -> (w597:bool)
        n247 = call <vilib>:"Edge Detector.vi"("Mode"=enum16{"Rising", "Falling", "Any"}."Rising", "Input"=w603) -> ("Output"=w594:bool)  [unwired: 9 in]
        n248 = call <vilib>:"Edge Detector.vi"("Mode"=enum16{"Rising", "Falling", "Any"}."Rising", "Input"=w597) -> ("Output"=w591:bool)  [unwired: 9 in]
        n249 = call <vilib>:"SR Flip Flop.vi"("Enable"=w594, "Reset"=w595, "Set"=w595) -> ("Output"=w593:bool)  [unwired: 8 in]
        n250 = call <vilib>:"SR Flip Flop.vi"("Enable"=w591, "Reset"=w592, "Set"=w592) -> ("Output"=w590:bool)  [unwired: 8 in]
        n251 = case shown="\"Initialize\", Default" w606 {
          selector: w606 -> [_ w626 w628]
          tunnel: [WPI_SolenoidValue."Off" ("Value") WPI_SolenoidValue."Off" ("Value") WPI_SolenoidValue."On" ("Value")] -> w589
          tunnel: [enum16{"Initialize", "Off", "On"}."Off" w625 w632] -> w602
          tunnel: w593 -> [_ w624 w630]
          frame "Initialize", Default {
          }
          frame "Off" {
            n252 = Select(t=enum16{"Initialize", "Off", "On"}."On", s=w624, f=w626) -> (s? t:f=w625:enum16{"Initialize", "Off", "On"})
          }
          frame "On" {
            n253 = Select(t=w628, s=w630, f=enum16{"Initialize", "Off", "On"}."Off") -> (s? t:f=w632:enum16{"Initialize", "Off", "On"})
          }
        }
        n254 = case shown="\"Initialize\", Default" w601 {
          selector: w601 -> [_ w614 w616]
          tunnel: [WPI_SolenoidValue."Off" ("Value") WPI_SolenoidValue."Off" ("Value") WPI_SolenoidValue."On" ("Value")] -> w599
          tunnel: [enum16{"Initialize", "Off", "On"}."Off" w613 w620] -> w596
          tunnel: w590 -> [_ w611 w618]
          frame "Initialize", Default {
          }
          frame "Off" {
            n255 = Select(t=enum16{"Initialize", "Off", "On"}."On", s=w611, f=w614) -> (s? t:f=w613:enum16{"Initialize", "Off", "On"})
          }
          frame "On" {
            n256 = Select(t=w616, s=w618, f=enum16{"Initialize", "Off", "On"}."Off") -> (s? t:f=w620:enum16{"Initialize", "Off", "On"})
          }
        }
        n257 = Wait (ms)(milliseconds to wait=u32 30) -> ()  [unwired: 1 out]
        n258 = call-poly <vilib>:"WPI_SolenoidSet.vi"("Value"=w589, "SolenoidDevRef"=w605) -> ()  [unwired: 8 in, 2 out]
        n259 = call-poly <vilib>:"WPI_SolenoidSet.vi"("Value"=w599, "SolenoidDevRef"=w600) -> ()  [unwired: 8 in, 2 out]
      }
    }
    frame Enabled {
    }
  }
  n260 = disable-structure shown="Disabled" {
    frame Disabled {
      n261 = call <vilib>:"WPI_SolenoidRefNum Registry Get.vi"("refnum name"="Lift") -> ("SolenoidDevRef"=w633:T28)  [unwired: 9 in, 1 out]
      n262 = while {
        tunnel: w633 -> [w636]
        stop <- FALSE stop-if-true
        w638 = TRUE ("Reset")
        n263 = global read "Robot Global Data.vi" "Share2"() -> (w643:bool)
        n264 = call <vilib>:"Edge Detector.vi"("Mode"=enum16{"Rising", "Falling", "Any"}."Rising", "Input"=w643) -> ("Output"=w639:bool)  [unwired: 9 in]
        n265 = call <vilib>:"SR Flip Flop.vi"("Enable"=w639, "Reset"=w638, "Set"=w638) -> ("Output"=w640:bool)  [unwired: 8 in]
        n266 = Wait (ms)(milliseconds to wait=u32 30) -> ()  [unwired: 1 out]
        n267 = Select(t=WPI_SolenoidValue."On" ("Value"), s=w640, f=WPI_SolenoidValue."Off" ("Value")) -> (s? t:f=w635:T31)
        n268 = call-poly <vilib>:"WPI_SolenoidSet.vi"("Value"=w635, "SolenoidDevRef"=w636) -> ()  [unwired: 8 in, 2 out]
      }
    }
    frame Enabled {
    }
  }
  n269 = call <vilib>:"CTRE_Phoenix_MotorControl_RefNumRegistryGet.vi"("refnum name"="Right1") -> ("PhoenixMotorControlDevRef"=w38:T20)  [unwired: 9 in, 1 out]
  n270 = call <vilib>:"CTRE_Phoenix_MotorControl_RefNumRegistryGet.vi"("refnum name"="Right2") -> ("PhoenixMotorControlDevRef"=w35:T20)  [unwired: 9 in, 1 out]
  n271 = call <vilib>:"CTRE_Phoenix_MotorControl_RefNumRegistryGet.vi"("refnum name"="Left2") -> ("PhoenixMotorControlDevRef"=w39:T20)  [unwired: 9 in, 1 out]
  n272 = call <vilib>:"CTRE_Phoenix_MotorControl_RefNumRegistryGet.vi"("refnum name"="Left1") -> ("PhoenixMotorControlDevRef"=w42:T20)  [unwired: 9 in, 1 out]
  n273 = call <vilib>:"ADIS16470 RefNum Registry Get.vi"("refnum name"="ADIS") -> ("data"=w26:T33)  [unwired: 9 in, 1 out]
  n274 = while {
    tunnel: w42 -> [w674]
    tunnel: w39 -> [w672]
    tunnel: w38 -> [w670]
    tunnel: w35 -> [w668]
    stop <- FALSE stop-if-true
    n275 = global read "Robot Global Data.vi" "DriveENCreset"() -> (w648:bool)
    n276 = call <vilib>:"Edge Detector.vi"("Mode"=enum16{"Rising", "Falling", "Any"}."Rising", "Input"=w648) -> ("Output"=w647:bool)  [unwired: 9 in]
    n277 = case shown="True" w647 {
      tunnel: w674 -> [w720 w731]
      tunnel: [w720 w730] -> w673
      tunnel: w672 -> [w719 w726]
      tunnel: [w719 w725] -> w671
      tunnel: w670 -> [w718 w724]
      tunnel: [w718 w723] -> w669
      tunnel: w668 -> [w717 w722]
      tunnel: [w717 w721] -> w667
      frame False {
      }
      frame True {
        n278 = call-poly <vilib>:"CTRE_Phoenix_MotorControl_SetIntegratedSensorPosition_TalonFX_Polymorphic.vi"("New Position"=0.0, "PhoenixMotorControlDevRef"=w731) -> ("PhoenixMotorControlDevRef"=w730:T20)  [unwired: 8 in, 1 out]
        n279 = call-poly <vilib>:"CTRE_Phoenix_MotorControl_SetIntegratedSensorPosition_TalonFX_Polymorphic.vi"("New Position"=0.0, "PhoenixMotorControlDevRef"=w724) -> ("PhoenixMotorControlDevRef"=w723:T20)  [unwired: 8 in, 1 out]
        n280 = call-poly <vilib>:"CTRE_Phoenix_MotorControl_SetIntegratedSensorPosition_TalonFX_Polymorphic.vi"("New Position"=0.0, "PhoenixMotorControlDevRef"=w726) -> ("PhoenixMotorControlDevRef"=w725:T20)  [unwired: 8 in, 1 out]
        n281 = call-poly <vilib>:"CTRE_Phoenix_MotorControl_SetIntegratedSensorPosition_TalonFX_Polymorphic.vi"("New Position"=0.0, "PhoenixMotorControlDevRef"=w722) -> ("PhoenixMotorControlDevRef"=w721:T20)  [unwired: 8 in, 1 out]
      }
    }
    n282 = call-poly <vilib>:"CTRE_Phoenix_MotorController_Get_TalonFX.vi"("PhoenixMotorControlDevRef"=w669) -> ("Position (Raw Sensor Units)"=w660:i32)  [unwired: 11 in, 3 out]
    n283 = call-poly <vilib>:"CTRE_Phoenix_MotorController_Get_TalonFX.vi"("PhoenixMotorControlDevRef"=w667) -> ("Position (Raw Sensor Units)"=w659:i32)  [unwired: 11 in, 3 out]
    n284 = call-poly <vilib>:"CTRE_Phoenix_MotorController_Get_TalonFX.vi"("PhoenixMotorControlDevRef"=w671) -> ("Position (Raw Sensor Units)"=w661:i32)  [unwired: 11 in, 3 out]
    n285 = call-poly <vilib>:"CTRE_Phoenix_MotorController_Get_TalonFX.vi"("PhoenixMotorControlDevRef"=w673) -> ("Position (Raw Sensor Units)"=w666:i32)  [unwired: 11 in, 3 out]
    n286 = Wait (ms)(milliseconds to wait=u32 10) -> ()  [unwired: 1 out]
    n287 = xnode "Inches/Count"("Wd"=4.0, "Sensor"=w660) -> ("Result"=w652:dbl)  [unwired: 1 in, 1 out]
    n288 = xnode "Inches/Count"("Wd"=4.0, "Sensor"=w666) -> ("Result"=w656:dbl)  [unwired: 1 in, 1 out]
    n289 = xnode "Inches/Count"("Wd"=4.0, "Sensor"=w661) -> ("Result"=w655:dbl)  [unwired: 1 in, 1 out]
    n290 = xnode "Inches/Count"("Wd"=4.0, "Sensor"=w659) -> ("Result"=w651:dbl)  [unwired: 1 in, 1 out]
    n291 = global write "Robot Global Data.vi" "Left1Enc"(w656) -> ()
    n292 = global write "Robot Global Data.vi" "Left2Enc"(w655) -> ()
    n293 = global write "Robot Global Data.vi" "Right1Enc"(w652) -> ()
    n294 = global write "Robot Global Data.vi" "Right2Enc"(w651) -> ()
    n295 = Add(x=w656, y=w655) -> (x+y=w658:dbl)
    n296 = Add(x=w652, y=w651) -> (x+y=w653:dbl)
    n297 = Divide(x=w658, y=2.0) -> (x/y=w650:dbl)
    n298 = Divide(x=w653, y=2.0) -> (x/y=w649:dbl)
    n299 = global write "Robot Global Data.vi" "LeftEncAvg"(w650) -> ()
    n300 = global write "Robot Global Data.vi" "RightEncAvg"(w649) -> ()
  }
  n301 = while {
    stop <- FALSE stop-if-true
    n302 = global read "Robot Global Data.vi" "RightEncAvg"() -> (w741:dbl)
    n303 = global read "Robot Global Data.vi" "LeftEncAvg"() -> (w736:dbl)
    n304 = global read "Robot Global Data.vi" "Pressure"() -> (w743:dbl)
    n305 = global read "Robot Global Data.vi" "TxAdj"() -> (w740:dbl)
    n306 = global read "Robot Global Data.vi" "Tx"() -> (w744:dbl)
    n307 = Number To Fractional String(number=w743) -> (F-format string=w755:string)  [unwired: 3 in]
    n308 = Number To Fractional String(number=w736) -> (F-format string=w756:string)  [unwired: 3 in]
    n309 = Number To Fractional String(number=w741) -> (F-format string=w757:string)  [unwired: 3 in]
    n310 = Number To Fractional String(number=w744) -> (F-format string=w758:string)  [unwired: 3 in]
    n311 = Number To Fractional String(number=w740) -> (F-format string=w759:string)  [unwired: 3 in]
    n312 = call-poly <vilib>:"NT Write Value.vi"("String"=w755, "Name"="DB/String 0") -> ()  [unwired: 9 in, 1 out]
    n313 = call-poly <vilib>:"NT Write Value.vi"("String"=w756, "Name"="DB/String 1") -> ()  [unwired: 9 in, 1 out]
    n314 = call-poly <vilib>:"NT Write Value.vi"("String"=w757, "Name"="DB/String 2") -> ()  [unwired: 9 in, 1 out]
    n315 = call-poly <vilib>:"NT Write Value.vi"("String"=w758, "Name"="DB/String 3") -> ()  [unwired: 9 in, 1 out]
    n316 = call-poly <vilib>:"NT Write Value.vi"("String"=w759, "Name"="DB/String 4") -> ()  [unwired: 9 in, 1 out]
    n317 = global read "Robot Global Data.vi" "Gyro Angle"() -> (w742:dbl)
    n318 = global read "Robot Global Data.vi" "ShooterVel"() -> (w739:dbl)
    n319 = global read "Robot Global Data.vi" "TDistance"() -> (w737:dbl)
    n320 = global read "Robot Global Data.vi" "Adjustment"() -> (w738:dbl)
    n321 = global read "Robot Global Data.vi" "AutoState"() -> (w767:string)
    n322 = Number To Fractional String(number=w742) -> (F-format string=w760:string)  [unwired: 3 in]
    n323 = Number To Fractional String(number=w739) -> (F-format string=w761:string)  [unwired: 3 in]
    n324 = Number To Fractional String(number=w737) -> (F-format string=w762:string)  [unwired: 3 in]
    n325 = Number To Fractional String(number=w738) -> (F-format string=w763:string)  [unwired: 3 in]
    n326 = call-poly <vilib>:"NT Write Value.vi"("String"=w760, "Name"="DB/String 5") -> ()  [unwired: 9 in, 1 out]
    n327 = call-poly <vilib>:"NT Write Value.vi"("String"=w761, "Name"="DB/String 6") -> ()  [unwired: 9 in, 1 out]
    n328 = call-poly <vilib>:"NT Write Value.vi"("String"=w762, "Name"="DB/String 7") -> ()  [unwired: 9 in, 1 out]
    n329 = call-poly <vilib>:"NT Write Value.vi"("String"=w763, "Name"="DB/String 8") -> ()  [unwired: 9 in, 1 out]
    n330 = call-poly <vilib>:"NT Write Value.vi"("String"=w767, "Name"="DB/String 9") -> ()  [unwired: 9 in, 1 out]
    n331 = Wait (ms)(milliseconds to wait=u32 50) -> ()  [unwired: 1 out]
    n332 = global read "Robot Global Data.vi" "Pressure"() -> (w733:dbl)
    n333 = call <vilib>:"WPI_DriverStationGet Alliance Info.vi"() -> ("Alliance"=w745:T43)  [unwired: 6 in, 5 out]
    n334 = global write "Robot Global Data.vi" "Alliance"(w745) -> ()
    n335 = Number To Fractional String(number=w733) -> (F-format string=w735:string)  [unwired: 3 in]
    n336 = call-poly <vilib>:"NT Write Value.vi"("String"=w735, "Name"="Pressure") -> ()  [unwired: 9 in, 1 out]
  }
  n337 = while {
    tunnel: w26 -> [w773]
    stop <- FALSE stop-if-true
    n338 = global read "Robot Global Data.vi" "GyroReset"() -> (w770:bool)
    n339 = call <vilib>:"Edge Detector.vi"("Mode"=enum16{"Rising", "Falling", "Any"}."Rising", "Input"=w770) -> ("Output"=w768:bool)  [unwired: 9 in]
    n340 = call <vilib>:"ADIS16470 Reset.vi"("Reset?"=w768, "ADIS16470DevRef"=w773) -> ("ADIS16470DevRef"=w774:T33)  [unwired: 8 in, 1 out]
    n341 = call <vilib>:"ADIS16470 Read.vi"("ADIS16470DevRef"=w774) -> ("ADIS16470 Value"=w772:T44)  [unwired: 7 in, 3 out]
    n342 = Unbundle By Name(w772) -> ("XAngle"=w771:dbl)
    n343 = global write "Robot Global Data.vi" "Gyro Angle"(w771) -> ()
    n344 = Wait (ms)(milliseconds to wait=u32 10) -> ()  [unwired: 1 out]
  }
  n345 = while {
    shift-right: [w808] -> _
    shift-left: _ -> [w805]
    shift-left: _ -> [w804]
    shift-left: _ -> [w803]
    shift-left: _ -> [w802]
    shift-left: _ -> [w801]
    shift-left: _ -> [w800]
    shift-left: _ -> [w799]
    shift-left: _ -> [w798]
    shift-left: _ -> [w806]
    shift-left: _ -> [w807]
    shift-right: [w793] -> _
    shift-left: _ -> [w792]
    shift-left: _ -> [w791]
    shift-left: _ -> [w790]
    shift-left: _ -> [w789]
    shift-left: _ -> [w788]
    shift-left: _ -> [w787]
    shift-left: _ -> [w786]
    shift-left: _ -> [w785]
    shift-left: _ -> [w784]
    shift-left: _ -> [w783]
    stop <- FALSE stop-if-true
    # "Camera Angle"
    # "RobotHeight"
    # "TargetHeight"
    n346 = Compound Arithmetic op=ADD(w792, w791, w790, w789, w788, w787, w786, w785, w784, w783) -> (w782:dbl)
    n347 = Compound Arithmetic op=ADD(w798, w799, w800, w801, w802, w803, w804, w805, w806, w807) -> (w797:dbl)
    n348 = Divide(x=w782, y=10.0) -> (x/y=w780:dbl)
    n349 = call-poly <vilib>:"NT Read Value.vi"("Name"="/limelight/ty") -> ("Numeric"=w816:dbl)  [unwired: 9 in, 1 out]
    n350 = call-poly <vilib>:"NT Read Value.vi"("Name"="/limelight/tx") -> ("Numeric"=w793:dbl)  [unwired: 9 in, 1 out]
    n351 = Divide(x=w797, y=10.0) -> (x/y=w795:dbl)
    n352 = global write "Robot Global Data.vi" "TDistance"(w795) -> ()
    n353 = Add(x=w816, y=22.5) -> (x+y=w811:dbl)
    n354 = global write "Robot Global Data.vi" "Ty"(w816) -> ()
    n355 = expression code="(x/180.0)*pi" "degrees to radians"(w811) -> (w815:dbl)
    n356 = expression code="(x/180.0)*pi" "degrees to radians"(w780) -> (w812:dbl)
    n357 = global write "Robot Global Data.vi" "Tx"(w780) -> ()
    n358 = call-poly <vilib>:"NT Read Value.vi"("Name"="/limelight/tv") -> ("Numeric"=w818:dbl)  [unwired: 9 in, 1 out]
    n359 = global write "Robot Global Data.vi" "Tv"(w818) -> ()
    n360 = xnode "Formula"("TH"=103.0 ("Output"), "Ty"=w815, "Tx"=w812, "RH"=28.0) -> ("Result"=w808:dbl)  [unwired: 1 in, 1 out]
    n361 = Wait (ms)(milliseconds to wait=u32 10) -> ()  [unwired: 1 out]
    n362 = call-poly <vilib>:"NT Write Value.vi"("Numeric"=0.0, "Name"="/limelight/camMode") -> ()  [unwired: 9 in, 1 out]
    n363 = call-poly <vilib>:"NT Write Value.vi"("Numeric"=0.0, "Name"="/limelight/ledMode") -> ()  [unwired: 9 in, 1 out]
    n364 = call-poly <vilib>:"NT Write Value.vi"("Numeric"=2.0, "Name"="/limelight/stream") -> ()  [unwired: 9 in, 1 out]
  }
  n365 = call <vilib>:"WPI_MotorControlRefNum Registry Get.vi"("refnum name"="LED") -> ("MotorControlDevRef"=w24:T20)  [unwired: 9 in, 1 out]
  n366 = while {
    shift-right: [w841] -> _
    shift-left: enum16{"wait", "init", "teleop", "auto", "end"}."init" -> [w842]
    tunnel: w24 -> [w845]
    tunnel: [w839] -> _
    stop <- FALSE stop-if-true
    n367 = global read "Robot Global Data.vi" "Robot Mode"() -> (w844:T45)
    n368 = global read "Robot Global Data.vi" "Alliance"() -> (w843:T43)
    n369 = case shown="\"wait\"" w842 {
      selector: w842 -> [w849 _ w872 w877 _]
      tunnel: [0.99 ("Motor Output") 0.99 ("Motor Output") w862 w874 -0.99 ("Motor Output")] -> w838
      tunnel: w844 -> [w850 _ _ w878 w889]
      tunnel: w843 -> [_ _ w868 w876 _]
      tunnel: [w847 enum16{"wait", "init", "teleop", "auto", "end"}."wait" w861 w875 w890] -> w841
      frame "wait" {
        n370 = Equal?(x=w850, y=WPI_DriverStationRobotMode2."Teleop Enabled" ("Robot Mode")) -> (x = y?=w853:bool)
        n371 = Equal?(x=w850, y=WPI_DriverStationRobotMode2."Autonomous Enabled" ("Robot Mode")) -> (x = y?=w856:bool)
        n372 = Select(t=enum16{"wait", "init", "teleop", "auto", "end"}."teleop", s=w853, f=w849) -> (s? t:f=w848:enum16{"wait", "init", "teleop", "auto", "end"})
        n373 = Select(t=enum16{"wait", "init", "teleop", "auto", "end"}."auto", s=w856, f=w848) -> (s? t:f=w847:enum16{"wait", "init", "teleop", "auto", "end"})
      }
      frame "init", Default {
      }
      frame "teleop" {
        # "Off"
        # "Blue"
        # "Red"
        n374 = call "Elapsed Time"() -> ("Time has Elapsed"=w860:bool)  [unwired: 12 in, 7 out]
        n375 = Equal?(x=WPI_DriverStationAllianceInfo."Red" ("Alliance"), y=w868) -> (x = y?=w870:bool)
        n376 = Equal?(x=WPI_DriverStationAllianceInfo."Blue" ("Alliance"), y=w868) -> (x = y?=w866:bool)
        n377 = Select(t=0.87 ("Motor Output"), s=w866, f=0.99 ("Motor Output")) -> (s? t:f=w863:dbl)
        n378 = Select(t=enum16{"wait", "init", "teleop", "auto", "end"}."end", s=w860, f=w872) -> (s? t:f=w861:enum16{"wait", "init", "teleop", "auto", "end"})
        n379 = Select(t=0.61 ("Motor Output"), s=w870, f=w863) -> (s? t:f=w862:dbl)
      }
      frame "auto" {
        n380 = case shown="\"Red\"" w876 {
          tunnel: [-0.09 ("Motor Output") -0.11 ("Motor Output") 0.99 ("Motor Output")] -> w874
          frame "Blue", Default {
          }
          frame "Red" {
          }
          frame "Invalid" {
          }
        }
        n381 = Equal?(x=w878, y=WPI_DriverStationRobotMode2."Teleop Enabled" ("Robot Mode")) -> (x = y?=w881:bool)
        n382 = Select(t=enum16{"wait", "init", "teleop", "auto", "end"}."teleop", s=w881, f=w877) -> (s? t:f=w875:enum16{"wait", "init", "teleop", "auto", "end"})
      }
      frame "end" {
        n383 = Equal?(x=w889, y=WPI_DriverStationRobotMode2."Autonomous Enabled" ("Robot Mode")) -> (x = y?=w887:bool)
        n384 = Select(t=enum16{"wait", "init", "teleop", "auto", "end"}."auto", s=w887, f=enum16{"wait", "init", "teleop", "auto", "end"}."end") -> (s? t:f=w890:enum16{"wait", "init", "teleop", "auto", "end"})
      }
    }
    n385 = call <vilib>:"WPI_MotorControlSetOutput.vi"("Output"=w838, "MotorControlDevRef"=w845) -> ()  [unwired: 7 in, 3 out]
    n386 = Wait (ms)(milliseconds to wait=u32 50) -> (millisecond timer value=w839:u32)
  }
  n387 = call <vilib>:"WPI_CompressorRefNum Registry Get.vi"("refnum name"="Compressor") -> ("CompressorDevRef"=w17:T46)  [unwired: 9 in, 1 out]
  n388 = while {
    tunnel: w17 -> [w898]
    stop <- FALSE stop-if-true
    w894 = TRUE ("Reset")
    n389 = global read "Robot Global Data.vi" "Share1"() -> (w896:bool)
    n390 = call <vilib>:"WPI_CompressorGetEnableState.vi"("CompressorDevRef"=w898) -> ("CompressorDevRef"=w892:T46, "Analog  Sensors"=w900:cluster{"Analog 0 (V)":dbl, "Analog 1 (V)":dbl})  [unwired: 4 in, 5 out]
    n391 = Unbundle(w900) -> ("Analog 0 (V)"=w899:dbl)  [unwired: 1 out]
    n392 = call <vilib>:"Edge Detector.vi"("Mode"=enum16{"Rising", "Falling", "Any"}."Rising", "Input"=w896) -> ("Output"=w895:bool)  [unwired: 9 in]
    n393 = global write "Robot Global Data.vi" "Pvolts"(w899) -> ()
    n394 = xnode "Formula 2"("Vsup"=4.8, "Vsen"=w899) -> ("Result"=w902:dbl)  [unwired: 1 in, 1 out]
    n395 = call <vilib>:"SR Flip Flop.vi"("Enable"=w895, "Reset"=w894, "Set"=w894) -> ("Output"=w897:bool)  [unwired: 8 in]
    n396 = global write "Robot Global Data.vi" "Pressure"(w902) -> ()
    n397 = case shown="False" w897 {
      tunnel: w892 -> [w905 w906]
      frame False {
        n398 = call <vilib>:"WPI_CompressorStart.vi"("CompressorDevRef"=w905) -> ()  [unwired: 9 in, 2 out]
      }
      frame True {
        n399 = call <vilib>:"WPI_CompressorStop.vi"("CompressorDevRef"=w906) -> ()  [unwired: 9 in, 2 out]
      }
    }
    n400 = Wait (ms)(milliseconds to wait=u32 50) -> ()  [unwired: 1 out]
  }
